vi "Station Wise Live Breakdown Status.vi"() -> ()   [LabVIEW 2017]
uses:
  Controls/Station_wise_live_breakdown_loop.ctl
  Controls/station_wise_loop_data.ctl
  <vilib>/addons/database/Connection.llb/Conn ObjectReference.ctl
  <vilib>/addons/database/Connection.llb/DB Tools Open Connec (Path).vi
  <vilib>/addons/database/Connection.llb/Conn Execute.vi
  <vilib>/addons/database/Recordset.llb/Rec Fetch Recordset Data (R).vi
  <vilib>/addons/database/Recordset.llb/Rec Destroy - Connection.vi
  Globle/Global 1.vi
  <vilib>/addons/database/NI_Database_API.lvlib
panel:
  out "ACTUAL  PLC COUNT":i32
  out "MACHINE 13":string
  out "Recipe Number":i32
  out "Product Code/":cluster{string, "ACTUAL  PLC COUNT":i32}[](array[cluster])
  out "Station Name":string[](array[string])
  out "Station Number":string[](array[string])
  out "Product List 2":string[][](array[string])
  out "appended path 2":path
  out "Product List":string[][](array[string])
  in  "Close":bool
  out "?":T1[](array[typedef])
  out "appended array":u32[](array[numeric])
  out "Table 2":string[][](array[string])
  out "String 2":string
  out "ACTUAL  PLC COUNT 2":i32
  out "ACTUAL  PLC PRODUCT CODE 2":i32
  out "Date / Time : 4":string
  out "String":string
  out "Table":string[][](array[string])
  out "Date / Time : 3":string
  out "ALARM ARRAY":string[](array[string])
  out "ALARAM CLST REF":bool
  out "String Indicator 8":bool
  out "Shift Time stamp":timestamp[](array[timestamp]) format="%<%X>T"
  in  "error in":errorcluster
  in  "Product code":string
  out "Production Count 7":i32
  in  "Rejection count 7":i32
  in  "Tab Control":T2(tab)
  out "Display 3":T3
  out "Display 1":T4
  out "Display 2":T3
  out "Display 4":T3
  out "Display 5":T3
  out "Display 6":T3
  out "Display 7":T3
  out "Display 8":T3
  out "Display 9":T3
  out "Display 10":T5
  out "MACHINE 12":cluster{"M1.1 8":bool, "M1.1 9":bool}
  out "MACHINE 11":string
  out "MACHINE 10":string
  out "MACHINE 8":string
  out "MACHINE 7":string
  out "MACHINE 6":string
  out "MACHINE 5":string
  out "MACHINE 4":string
  out "MACHINE 3":string
  out "MACHINE 2":string
  out "MACHINE 1":string
  out "MACHINE 8":T6
  out "MACHINE 7":T6
  out "MACHINE 6":T6
  out "MACHINE 5":T6
  out "MACHINE 4":T6
  out "MACHINE 3":T6
  out "MACHINE 2":T6
  out "Autonomous Check Points Press":T7
  out "MACHINE 1":T6
  out "MACHINE 9":T6
  out "MACHINE 10":T6
  out "Autonomous Check Points Oven":cluster{"ALARAM 1":bool}
  out "OVEN STATUS AUTONOMOUS":T8
  out "10":T9 caption="500T-1345678998uiyfghbu" {"PRESSURE_2nd" format="%#_g bar"; "PRESSURE_1st" format="%#_g bar"; "HOLDING_TIME" format="%#_g Sec"; "MR_RETURN_TIME" format="%#_g Sec"}
  out "9":T9 caption="500T-1" {"PRESSURE_2nd" format="%#_g bar"; "PRESSURE_1st" format="%#_g bar"; "HOLDING_TIME" format="%#_g Sec"; "MR_RETURN_TIME" format="%#_g Sec"}
  out "8":T9 caption="400T-4" {"PRESSURE_2nd" format="%#_g bar"; "PRESSURE_1st" format="%#_g bar"; "HOLDING_TIME" format="%#_g Sec"; "MR_RETURN_TIME" format="%#_g Sec"}
  out "6":T9 caption="250T-3" {"PRESSURE_2nd" format="%#_g bar"; "PRESSURE_1st" format="%#_g bar"; "HOLDING_TIME" format="%#_g Sec"; "MR_RETURN_TIME" format="%#_g Sec"}
  out "5":T9 caption="400T-1" {"PRESSURE_2nd" format="%#_g bar"; "PRESSURE_1st" format="%#_g bar"; "HOLDING_TIME" format="%#_g Sec"; "MR_RETURN_TIME" format="%#_g Sec"}
  out "4":T9 caption="400T-2" {"PRESSURE_2nd" format="%#_g bar"; "PRESSURE_1st" format="%#_g bar"; "HOLDING_TIME" format="%#_g Sec"; "MR_RETURN_TIME" format="%#_g Sec"}
  out "1":T9 caption="150T-1" {"PRESSURE_2nd" format="%#_g bar"; "PRESSURE_1st" format="%#_g bar"; "HOLDING_TIME" format="%#_g Sec"; "MR_RETURN_TIME" format="%#_g Sec"}
  out "2":T9 caption="250T-2" {"PRESSURE_2nd" format="%#_g bar"; "PRESSURE_1st" format="%#_g bar"; "HOLDING_TIME" format="%#_g Sec"; "MR_RETURN_TIME" format="%#_g Sec"}
  out "3":T9 caption="400T-3" {"PRESSURE_2nd" format="%#_g bar"; "PRESSURE_1st" format="%#_g bar"; "HOLDING_TIME" format="%#_g Sec"; "MR_RETURN_TIME" format="%#_g Sec"}
  out "7":T9 caption="250T-4" {"PRESSURE_2nd" format="%#_g bar"; "PRESSURE_1st" format="%#_g bar"; "HOLDING_TIME" format="%#_g Sec"; "MR_RETURN_TIME" format="%#_g Sec"}
  out "1 5":T10 caption="400T-4 OVEN" {"Heating_time" format="%#_g Sec"; "Bottom_zone_8" format="%#_g °C"; "Bottom_zone_7" format="%#_g °C"; "Bottom_zone_6" format="%#_g °C"; "Bottom_zone_5" format="%#_g °C"; "Bottom_zone_4" format="%#_g °C"; "Bottom_zone_3" format="%#_g °C"; "Bottom_zone_2" format="%#_g °C"; "Bottom_zone_1" format="%#_g °C"; "Top_zone_8" format="%#_g °C"; "Top_zone_7" format="%#_g °C"; "Top_zone_6" format="%#_g °C"; "Top_zone_5" format="%#_g °C"; "Top_zone_4" format="%#_g °C"; "Top_zone_3" format="%#_g °C"; "Top_zone_2" format="%#_g °C"; "Top_zone_1" format="%#_g °C"}
  out "1 4":T10 caption="400T-3 OVEN" {"Heating_time" format="%#_g Sec"; "Bottom_zone_8" format="%#_g °C"; "Bottom_zone_7" format="%#_g °C"; "Bottom_zone_6" format="%#_g °C"; "Bottom_zone_5" format="%#_g °C"; "Bottom_zone_4" format="%#_g °C"; "Bottom_zone_3" format="%#_g °C"; "Bottom_zone_2" format="%#_g °C"; "Bottom_zone_1" format="%#_g °C"; "Top_zone_8" format="%#_g °C"; "Top_zone_7" format="%#_g °C"; "Top_zone_6" format="%#_g °C"; "Top_zone_5" format="%#_g °C"; "Top_zone_4" format="%#_g °C"; "Top_zone_3" format="%#_g °C"; "Top_zone_2" format="%#_g °C"; "Top_zone_1" format="%#_g °C"}
  out "1 3":T10 caption="400T-2 OVEN" {"Heating_time" format="%#_g Sec"; "Bottom_zone_8" format="%#_g °C"; "Bottom_zone_7" format="%#_g °C"; "Bottom_zone_6" format="%#_g °C"; "Bottom_zone_5" format="%#_g °C"; "Bottom_zone_4" format="%#_g °C"; "Bottom_zone_3" format="%#_g °C"; "Bottom_zone_2" format="%#_g °C"; "Bottom_zone_1" format="%#_g °C"; "Top_zone_8" format="%#_g °C"; "Top_zone_7" format="%#_g °C"; "Top_zone_6" format="%#_g °C"; "Top_zone_5" format="%#_g °C"; "Top_zone_4" format="%#_g °C"; "Top_zone_3" format="%#_g °C"; "Top_zone_2" format="%#_g °C"; "Top_zone_1" format="%#_g °C"}
  out "1 2":T10 caption="400T-1 OVEN" {"Heating_time" format="%#_g Sec"; "Bottom_zone_8" format="%#_g °C"; "Bottom_zone_7" format="%#_g °C"; "Bottom_zone_6" format="%#_g °C"; "Bottom_zone_5" format="%#_g °C"; "Bottom_zone_4" format="%#_g °C"; "Bottom_zone_3" format="%#_g °C"; "Bottom_zone_2" format="%#_g °C"; "Bottom_zone_1" format="%#_g °C"; "Top_zone_8" format="%#_g °C"; "Top_zone_7" format="%#_g °C"; "Top_zone_6" format="%#_g °C"; "Top_zone_5" format="%#_g °C"; "Top_zone_4" format="%#_g °C"; "Top_zone_3" format="%#_g °C"; "Top_zone_2" format="%#_g °C"; "Top_zone_1" format="%#_g °C"}
  out "1 8":T11 caption="500T-1 OVEN" {"Bottom Zone\ntemperature" format="%#_g °C"; "Heating_time" format="%#_g Sec"; "Top Zone\ntemperature" format="%#_g °C"}
  out "1 7":T12 caption="250T-1 OVEN" {"Heating_time" format="%#_g Sec"; "Bottom_zone_3" format="%#_g °C"; "Bottom_zone_2" format="%#_g °C"; "Bottom_zone_1" format="%#_g °C"; "Top_zone_3" format="%#_g °C"; "Top_zone_2" format="%#_g °C"; "Top_zone_1" format="%#_g °C"}
  out "1 6":T10 caption="400T-5 OVEN" {"Heating_time" format="%#_g Sec"; "Bottom_zone_8" format="%#_g °C"; "Bottom_zone_7" format="%#_g °C"; "Bottom_zone_6" format="%#_g °C"; "Bottom_zone_5" format="%#_g °C"; "Bottom_zone_4" format="%#_g °C"; "Bottom_zone_3" format="%#_g °C"; "Bottom_zone_2" format="%#_g °C"; "Bottom_zone_1" format="%#_g °C"; "Top_zone_8" format="%#_g °C"; "Top_zone_7" format="%#_g °C"; "Top_zone_6" format="%#_g °C"; "Top_zone_5" format="%#_g °C"; "Top_zone_4" format="%#_g °C"; "Top_zone_3" format="%#_g °C"; "Top_zone_2" format="%#_g °C"; "Top_zone_1" format="%#_g °C"}
  out "error out":errorcluster
  # "CLUSTER REFRENCE"
  # "Station Wise Live Status"
  # "Communication"
  # "1st screen\n\n5 10.0.0.73\n4 10.0.0.71\n3 10.0.0.69\n7 10.0.0.61"
  # "2nd Screen\n\n8 10.0.0.63\n9 10.0.0.75\n1 10.0.0.67"
  # "Safety"
  # "Startup/Setup"
  # "1236 684"
  # "500t1 ,250-2,400-3,400-2,400-1,250-3,400-4,400-5---> PRESS\n400-1,400-2,400-3,400-4,400-5,250-1,500-1--->OVEN"
  # "1366*768"
  # "500t1 ,250-2,  400-3,400-2,400-1,250-3,400-4,400-5   ,  NA   ---> PRESS\n500-1,    NA,   400-3,400-2,400-1,   NA,    400-4,400-5, 250-1--->OVEN"
  # "Raw Material Not Available"
  # "Under Maintenance"
  # "Under Quality Review"
  # "Parameter OutOff Range"
  # "Production Recording System"
  # "Machine Under Maintanance"
  # "Product Name"
  # "Product Name"
  # "Product Name"
  # "Product Name"
  # "Product Name"
  # "Product Name"
  # "Production Recording System"
  # "Machine Under Maintanance"
  # "Product Name"
  # "Product Name"
  # "Product Name"
  # "Communication:-"
  # "Autonomous Maintanence Checksheet"
  # "T.F. Process Parameter Monitoring"
  # "Oven Process Parameter Monitoring"
  # "Machine Under Maintanance"
  # "Oven Process Parameter Monitoring"
  # "Machine Under Maintanance"
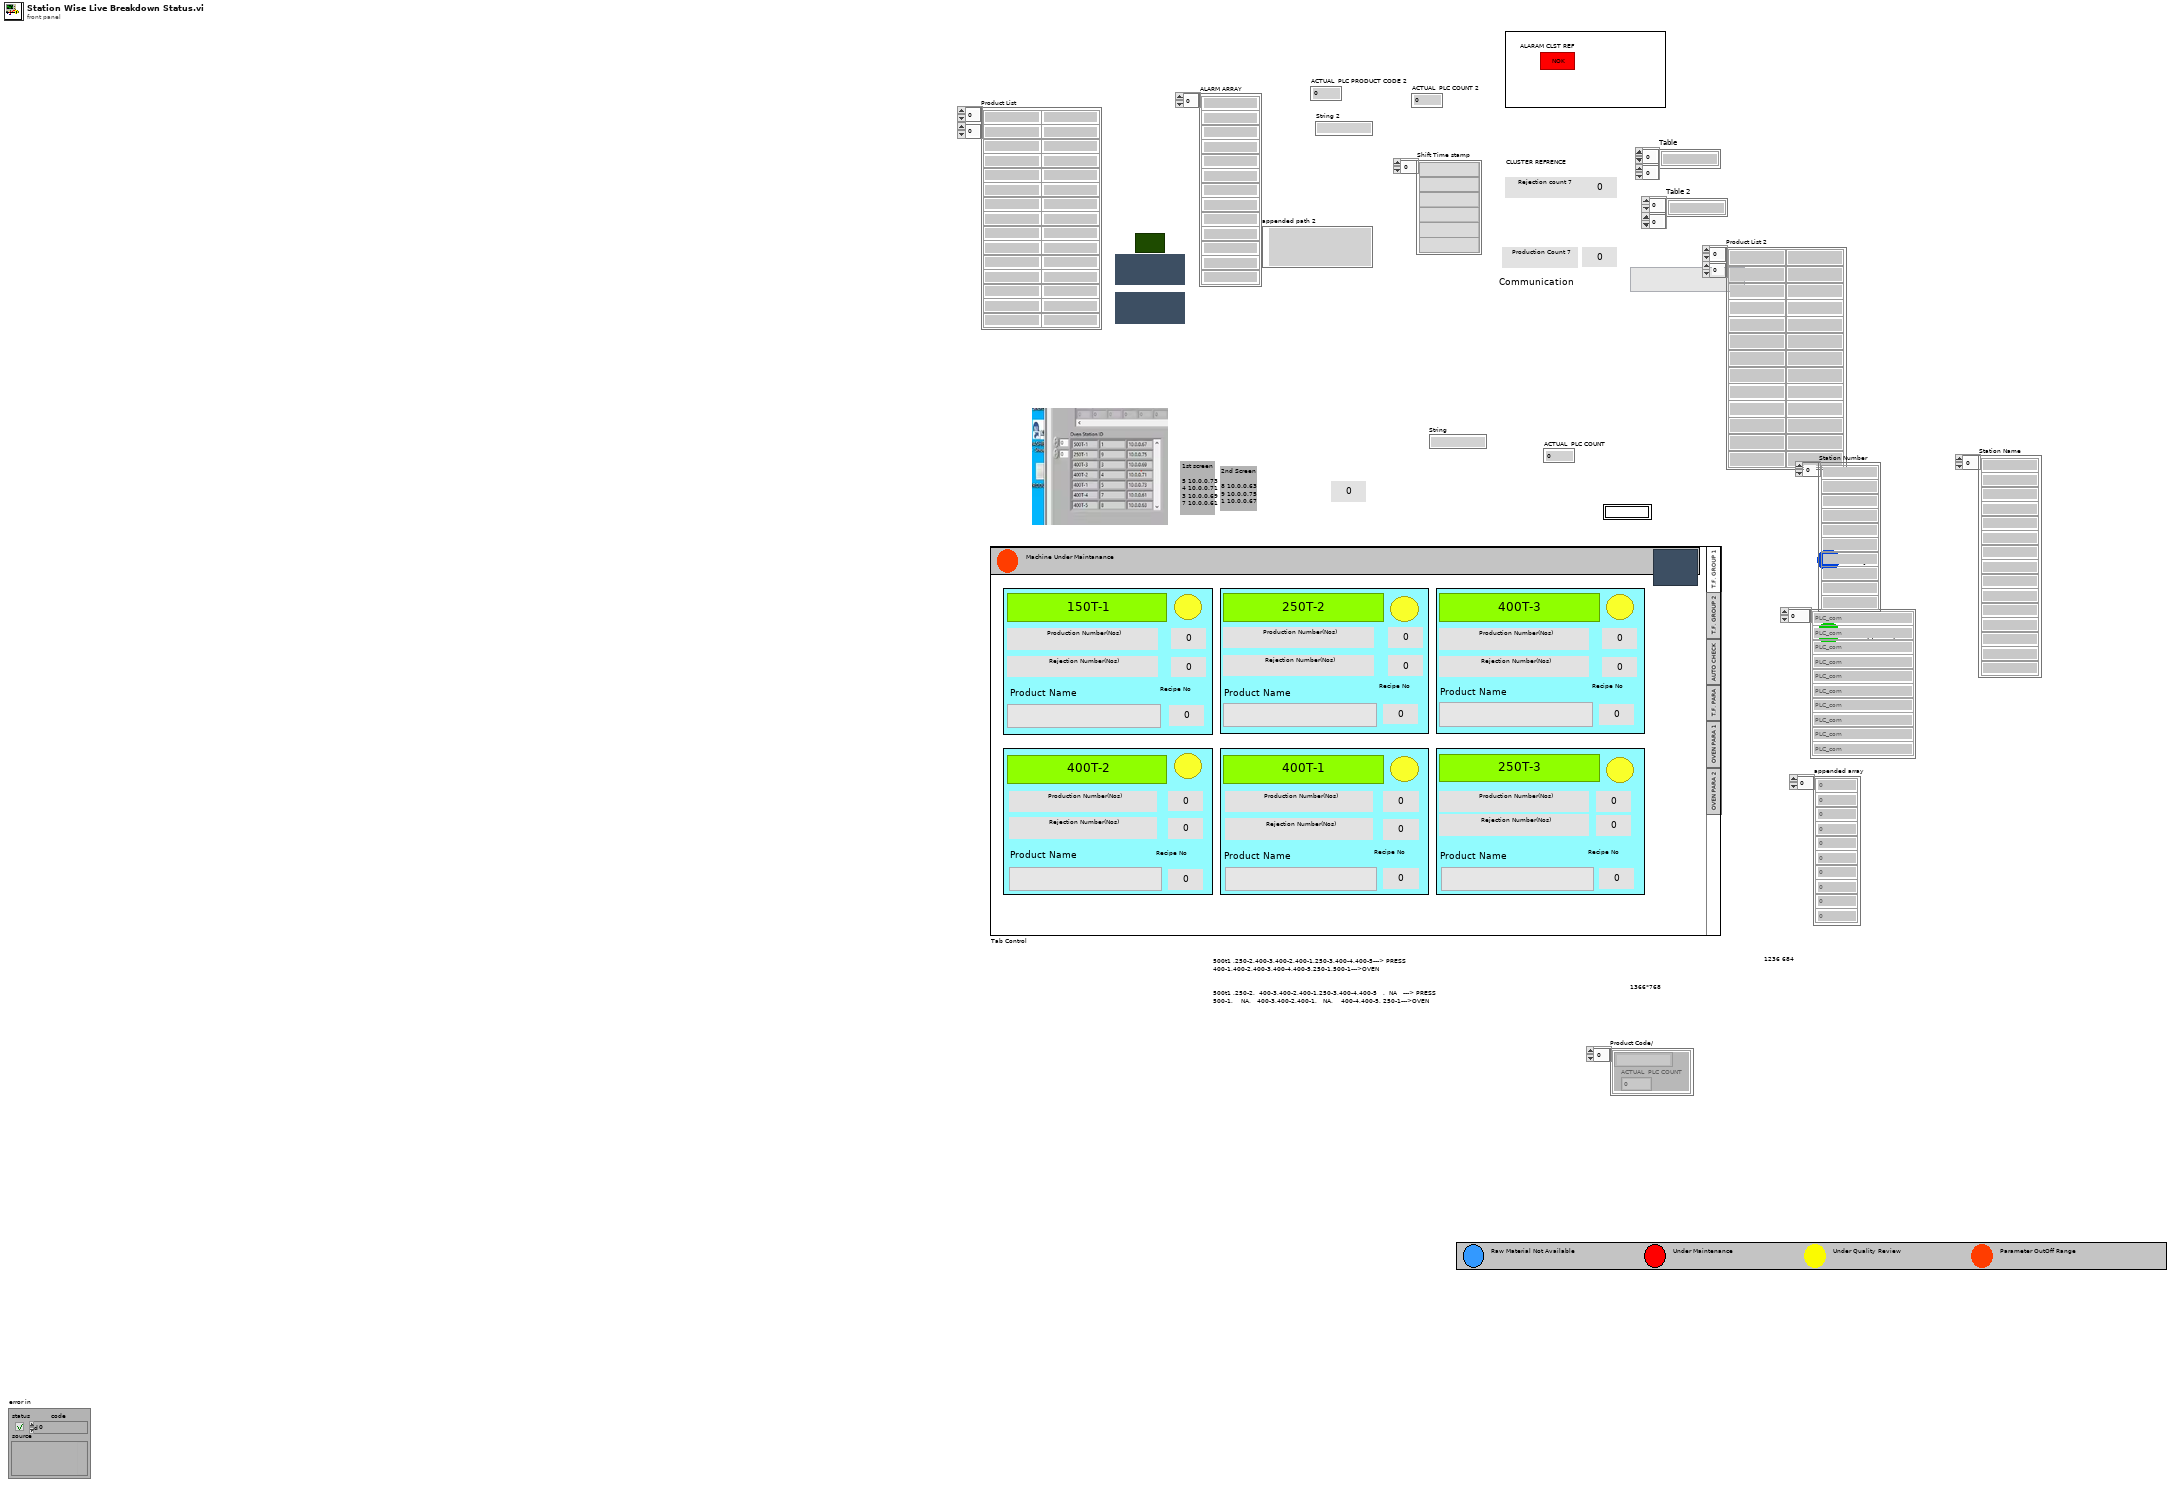
[diagram p1: front panel]
types:
  T1 = typedef "Station_wise_live_breakdown_loop.ctl" = enum16{"Int_3", "Break_down", "Rejection_count", "STOP", "BUTTON_SWITCH", "Init_2", "Alaram_stat", "Product_count", "PLC_com", "Init", "Oven_Reading"}
  T2 = enum32{"T.F. GROUP 1", "T.F. GROUP 2", "AUTO CHECK", "T.F. PARA", "OVEN PARA 1", "OVEN PARA 2"}
  T3 = cluster{"Status 10":cluster{"S":bool, "l":bool, "M":bool, "Q":bool, "P":bool}, "Station 3":bool, "Production Number(Nos)":i32, "Rejection Number(Nos)":i32, "Press COM 1":bool, "Product code 10":string, "Recipe No":i32}
  T4 = cluster{"Status 10":cluster{"S":bool, "l":bool, "M":bool, "Q":bool, "P":bool}, "Station Name":bool, "Production Number(Nos)":i32, "Rejection Number(Nos)":i32, "Press COM 1":bool, "Product code 10":string, "Recipe No":i32}
  T5 = cluster{"Status 10":cluster{"S":bool, "l":bool, "M":bool, "Q":bool, "P":bool}, "Station 3":bool, "Production\nCount 3":i32, "Rejection count 3":i32, "String Indicator 3":bool, "Product code 10":string}
  T6 = cluster{"M1.1":bool, "M1.1 2":bool, "M1.1 3":bool, "M1.1 4":bool, "M1.1 5":bool, "M1.1 6":bool, "M1.1 7":bool, "M1.1 8":bool, "M1.1 9":bool}
  T7 = cluster{"ALARAM 1":bool, "ALARAM 2":bool, "ALARAM 3":bool, "ALARAM 4":bool, "ALARAM 5":bool, "ALARAM 6":bool, "ALARAM 7":bool}
  T8 = cluster{"500T-1":bool, "M1.1 7":bool, "400T-3":bool, "400T-2":bool, "400T-1":bool, "M1.1 7":bool, "M1.1 6":bool, "M1.1 10":bool, "M1.1 11":bool}
  T9 = cluster{"MR_RETURN_TIME":dbl, "HOLDING_TIME":dbl, "PRESSURE_1st":dbl, "PRESSURE_2nd":dbl}
  T10 = cluster{"400T-2 OVEN COM":bool, "Station Name 2":bool, "Top_zone_1":dbl, "Top_zone_2":dbl, "Top_zone_3":dbl, "Top_zone_4":dbl, "Top_zone_5":dbl, "Top_zone_6":dbl, "Top_zone_7":dbl, "Top_zone_8":dbl, "Bottom_zone_1":dbl, "Bottom_zone_2":dbl, "Bottom_zone_3":dbl, "Bottom_zone_4":dbl, "Bottom_zone_5":dbl, "Bottom_zone_6":dbl, "Bottom_zone_7":dbl, "Bottom_zone_8":dbl, "Heating_time":dbl}
  T11 = cluster{"400T-2 OVEN COM":bool, "Station Name 2":bool, "Top Zone\ntemperature":dbl, "Bottom Zone\ntemperature":dbl, "Heating_time":dbl}
  T12 = cluster{"400T-2 OVEN COM":bool, "Station Name 2":bool, "Top_zone_1":dbl, "Top_zone_2":dbl, "Top_zone_3":dbl, "Bottom_zone_1":dbl, "Bottom_zone_2":dbl, "Bottom_zone_3":dbl, "Heating_time":dbl}
  T13 = typedef "station_wise_loop_data.ctl" = cluster{"Product List":string[][], "SQL reference":T14, "Indicator refrence":refnum<vi>[], "Station Number":string[], "Shift Time stamp":timestamp[], "Com Status Station":string[], "ALARAM INDICATOR REF":refnum<vi>[], "Reading":refnum<vi>[], "Read Parameteres":string[][], "Station Name":string[], "Oven Read Parameteres":string[][]}
  T14 = typedef "NI_Database_API.lvlib/Conn ObjectReference.ctl" = refnum<k1>
  T15 = enum32{"invalid app kind", "Development System", "Run Time System", "Student Edition", "Embedded LabVIEW", "Evaluation", "Custom"}
  T16 = typedef "NI_Database_API.lvlib/Rec ObjectReference.ctl" = refnum<k1>
  T17 = enum32{"T.F. GROUP 1", "T.F. GROUP 2", "AUTO CHECK", "T.F. PARA", "OVEN PARA 1", "OVEN PARA 2"}[]
  T18 = cluster{"[0]":dbl, "[1]":dbl, "[2]":dbl, "[3]":dbl}
  T19 = cluster{"[0]":bool, "[1]":bool, "[2]":bool, "[3]":bool, "[4]":bool}
  T20 = cluster{"array[0]":bool, "array[1]":bool, "array[2]":bool, "array[3]":bool, "array[4]":bool}
  T21 = cluster{"[0]":bool, "[1]":bool, "[2]":bool, "[3]":bool, "[4]":bool, "[5]":bool, "[6]":bool, "[7]":bool, "[8]":bool}
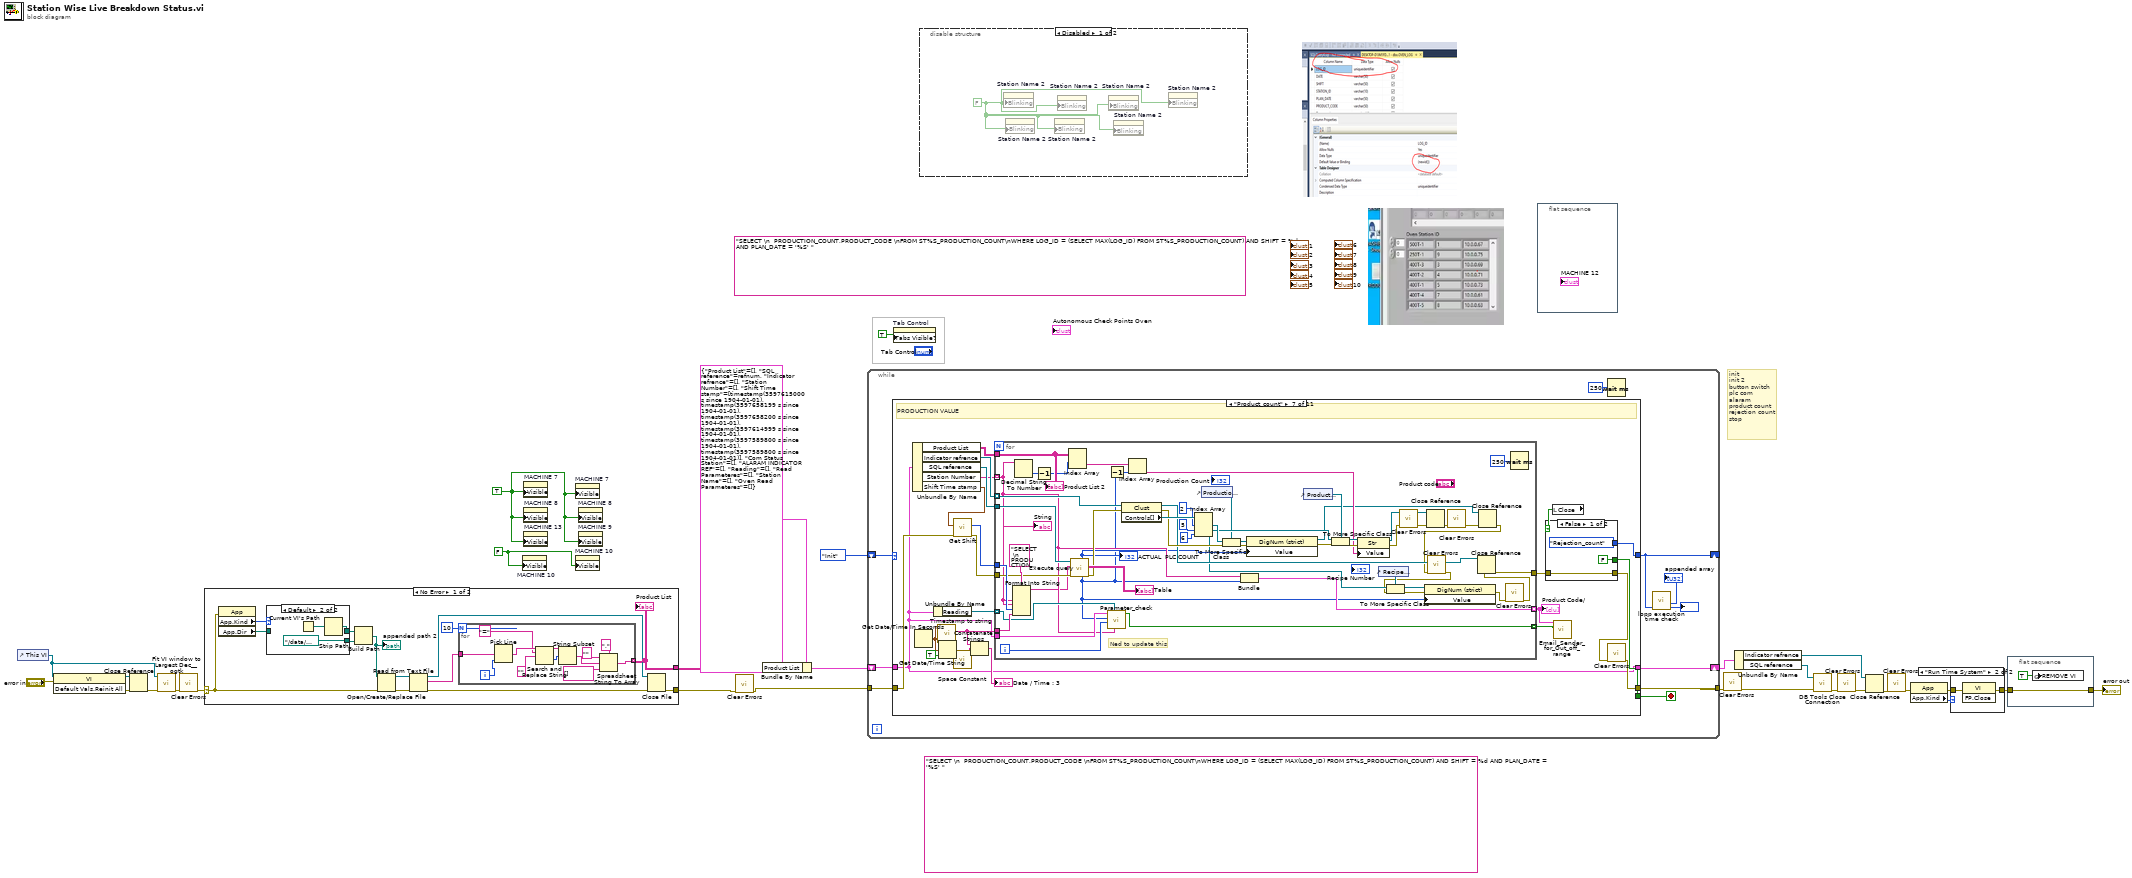
[diagram p0: block diagram]
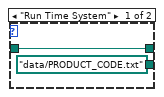
[diagram p4: hidden frame]
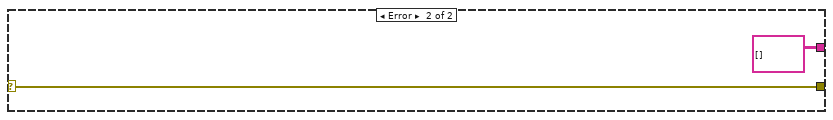
[diagram p5: hidden frame]
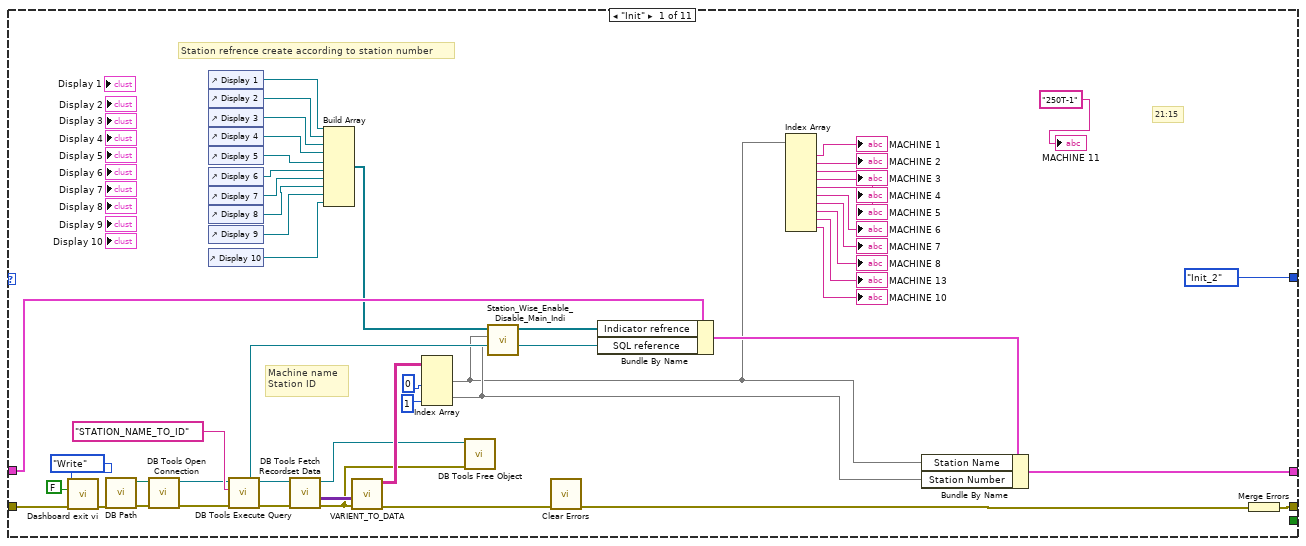
[diagram p6: hidden frame]
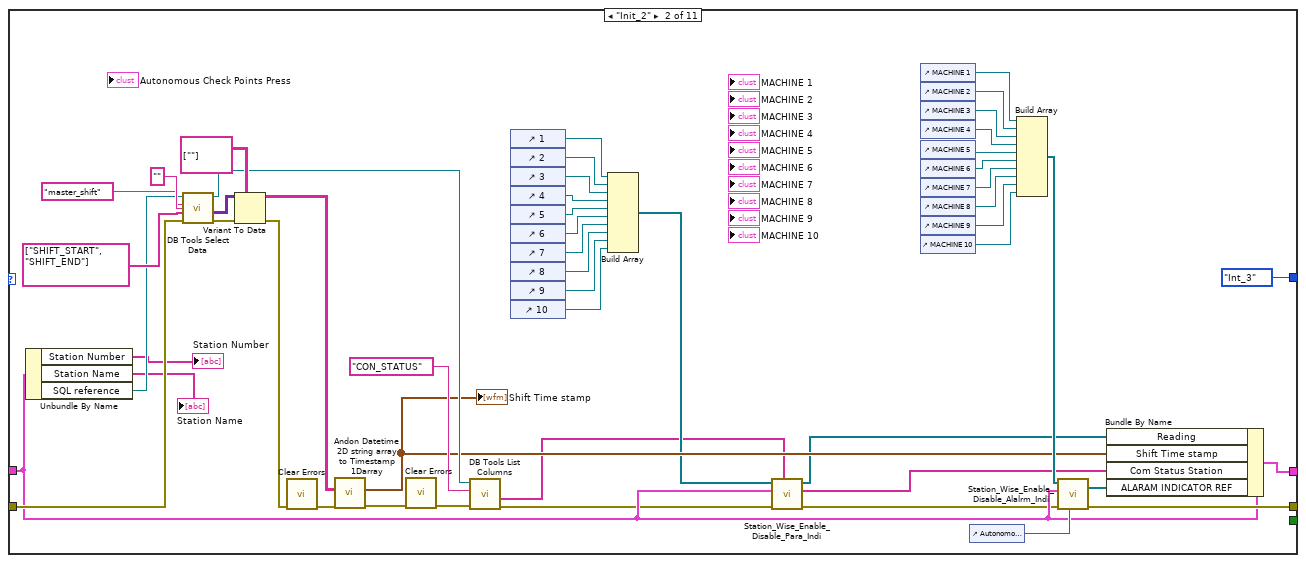
[diagram p7: hidden frame]
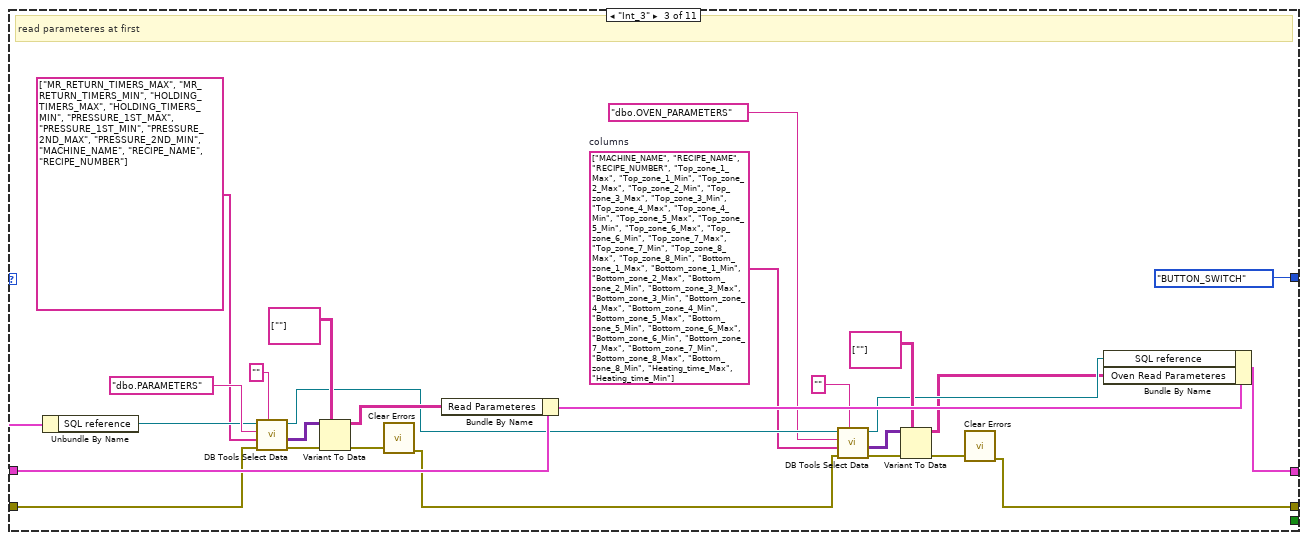
[diagram p8: hidden frame]
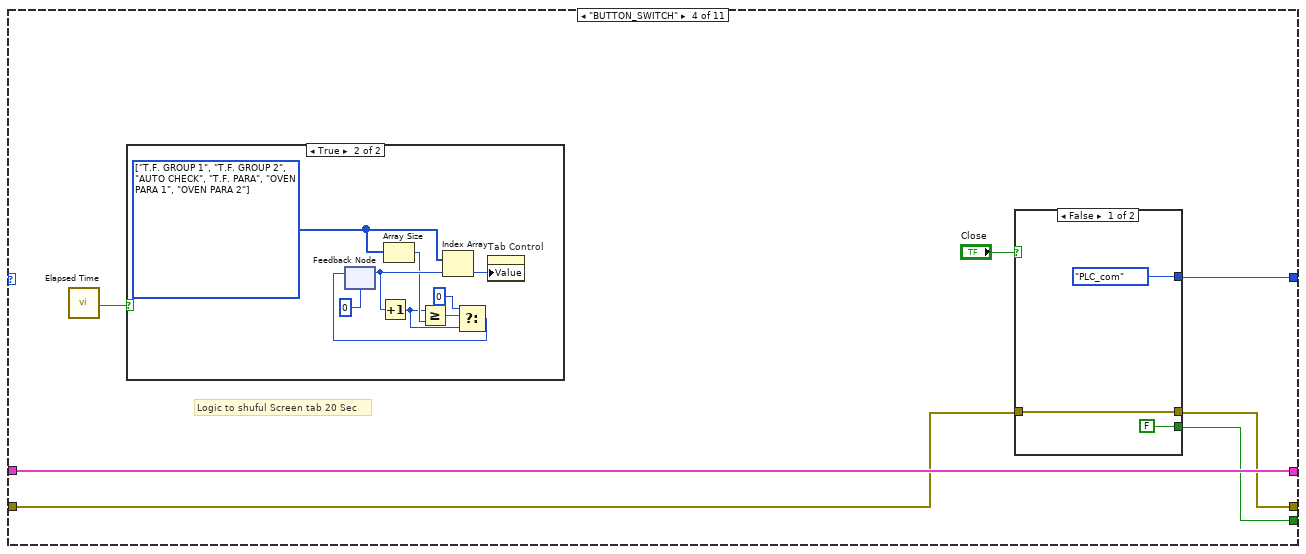
[diagram p9: hidden frame]
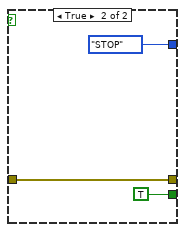
[diagram p11: hidden frame]
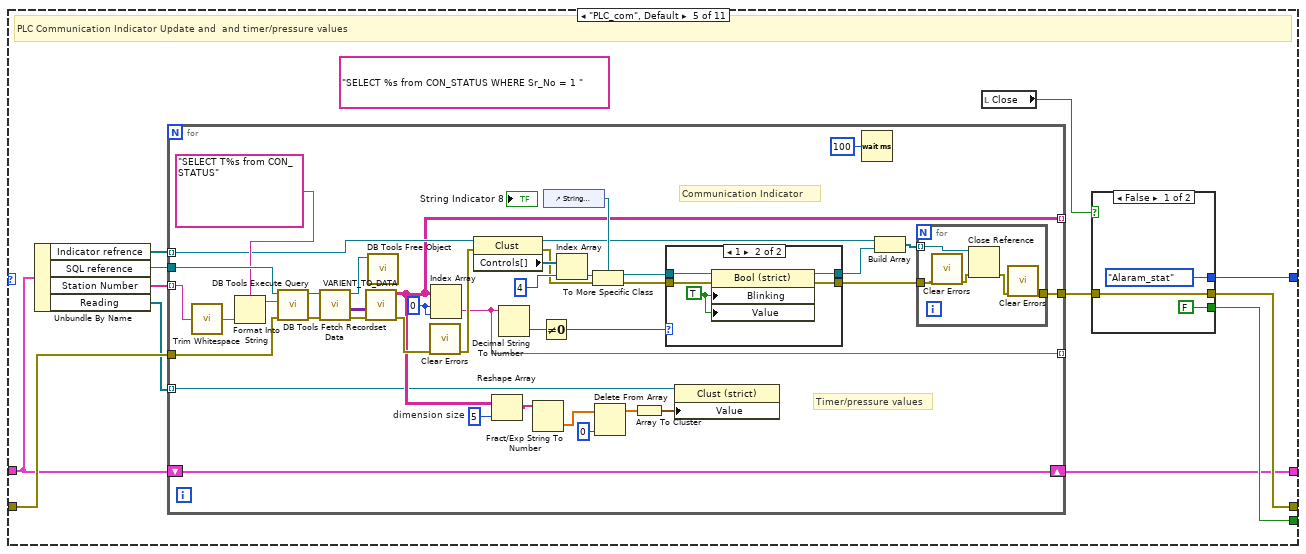
[diagram p12: hidden frame]
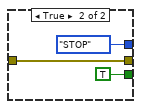
[diagram p13: hidden frame]
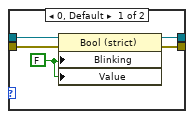
[diagram p14: hidden frame]
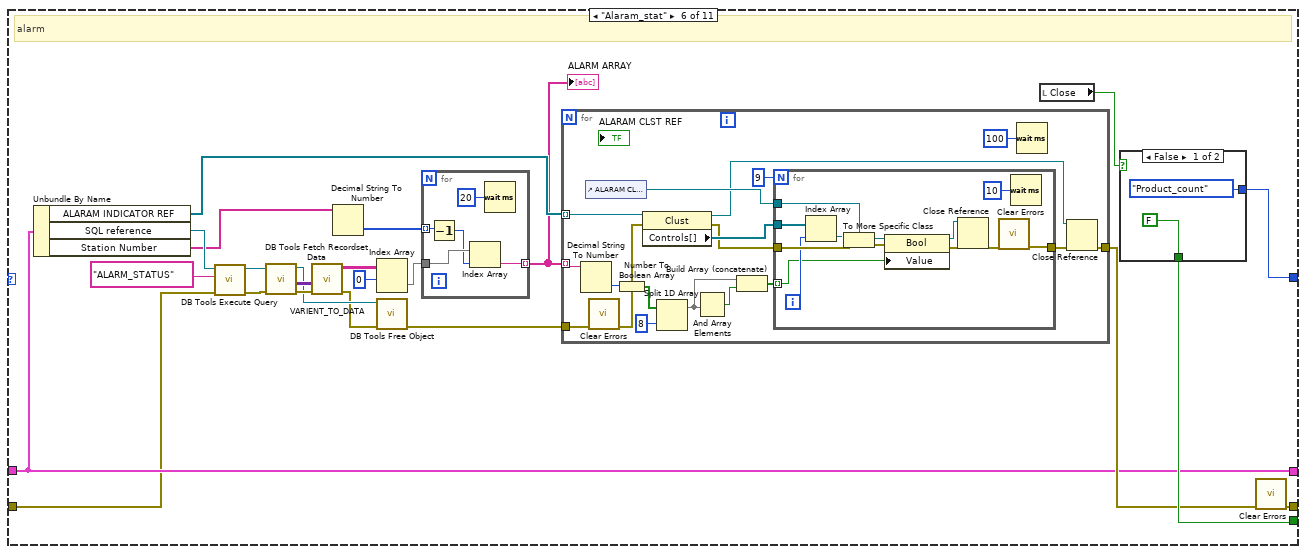
[diagram p15: hidden frame]
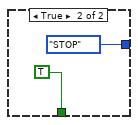
[diagram p16: hidden frame]
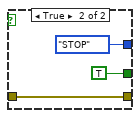
[diagram p17: hidden frame]
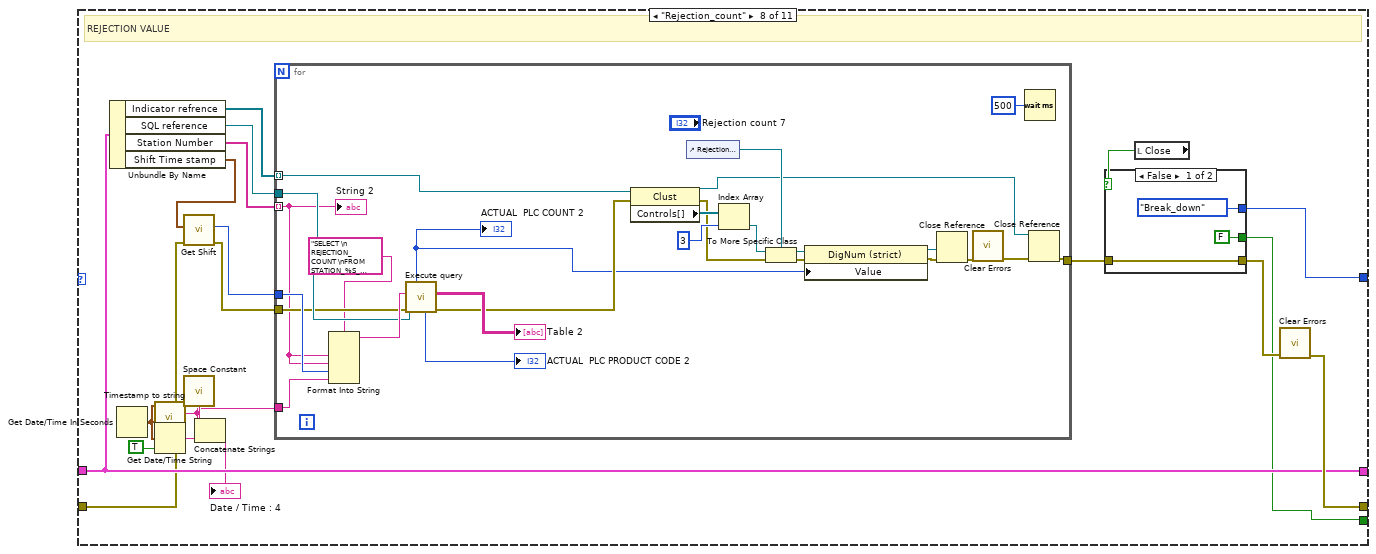
[diagram p18: hidden frame]
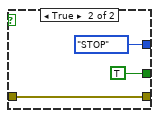
[diagram p19: hidden frame]
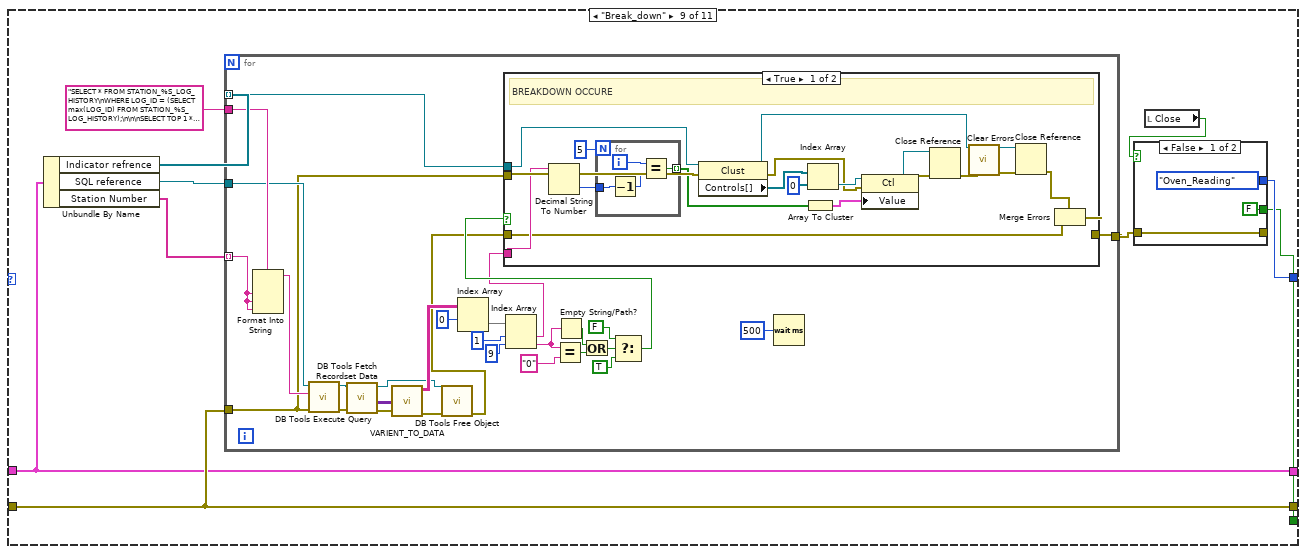
[diagram p20: hidden frame]
diagram:
  (unwired) "SELECT \n  PRODUCTION_COUNT,PRODUCT_CODE \nFROM ST%S_PRODUCTION_COUNT\nWHERE LOG_ID = (SELECT MAX(LOG_ID) FROM ST%S_PRODUCTION_COUNT) AND SHIFT = %d AND PLAN_DATE = '%S' " ("SQL query")
  (unwired) "SELECT \n  PRODUCTION_COUNT,PRODUCT_CODE \nFROM ST%S_PRODUCTION_COUNT\nWHERE LOG_ID = (SELECT MAX(LOG_ID) FROM ST%S_PRODUCTION_COUNT) AND SHIFT = %d AND PLAN_DATE = '%S' " ("SQL query")
  w5 = FALSE
  w19 = TRUE
  # "init\ninit 2\nbutton switch\nplc com\nalaram\nproduct count\nrejection count\nstop"
  n1 = control-ref of="This VI"() -> (w2:refnum<vi>)
  n2 = invoke class="VI" method="Default Vals.Reinit All"(reference=w2, error in="error in") -> (reference out=w8:refnum<vi>, error out=w7:errorcluster)  [unwired: 1 in, 1 out]
  n3 = Close Reference(reference=w8, error in (no error)=w7) -> (error out=w4:errorcluster)
  n4 = call <userlib>:"Fit VI window to Largest Dec__ogtk.vi"("error in (no error)"=w4, "VI Ref (calling VI)"=w2) -> ("error out"=w3:errorcluster)  [unwired: 4 in, 1 out]
  n5 = call <vilib>:"Clear Errors.vi"("error in (no error)"=w3) -> ("error out"=w1:errorcluster)  [unwired: 5 in, 1 out]
  n6 = case shown="No Error" w1 {
    selector: w1 -> [w30 w62]
    tunnel: [w34 w62] -> w10
    tunnel: [w31 string[][] [] ("delimiter (Tab)")] -> w28
    frame No Error {
      n7 = property class="App"(error in=w30) -> ("App.Kind"=w43:T15, "App.Dir"=w42:path)  [unwired: 1 in, 2 out]
      n8 = case shown="Default" w43 {
        tunnel: w42 -> [w57 _]
        tunnel: [path "data/PRODUCT_CODE.txt" ("path") path "../data/PRODUCT_CODE.txt" ("path")] -> w40
        tunnel: [w57 w58] -> w39
        frame "Run Time System" {
        }
        frame Default {
          n9 = Current VI's Path() -> (path=w59:path)
          n10 = Strip Path(path=w59) -> (stripped path=w58:path)  [unwired: 1 out]
        }
      }
      n11 = Build Path(base path=w39, name or relative path=w40) -> (appended path=w41:path)
      "appended path 2" <- w41
      n12 = Open/Create/Replace File(file path (use dialog)=w41, error in=w30) -> (refnum out=w38:refnum<file>, error out=w37:errorcluster)  [unwired: 4 in, 1 out]
      n13 = Read from Text File(file (use dialog)=w38, error in=w37) -> (refnum out=w35:refnum<file>, text=w33:string, error out=w36:errorcluster)  [unwired: 2 in, 1 out]
      n14 = for {
        N: 10 -> [_]
        tunnel: w33 -> [w46]
        tunnel: [w44] -> w31 mode=indexing
        i -> [w47]
        n15 = Pick Line(multi-line string=w46, line index=w47) -> (output string=w48:string)  [unwired: 1 in]
        n16 = Search and Replace String(input string=w48, search string="=" ("format string"), replace string="" ("search string")) -> (result string=w50:string, offset past replacement=w51:i32)  [unwired: 5 in, 2 out]
        n17 = String Subset(string=w50, offset (0)=w51) -> (substring=w49:string)  [unwired: 1 in]
        n18 = Spreadsheet String To Array(delimiter (Tab)=",", format string="", spreadsheet string=w49, array type (2D Dbl)=string[] [] ("delimiter (Tab)")) -> (array=w44:string[])
      }
      "Product List" <- w31
      n19 = Close File(refnum=w35, error in=w36) -> (error out=w34:errorcluster)  [unwired: 1 out]
    }
    frame Error {
    }
  }
  n20 = property on="MACHINE 10" class="Str"("Visible"=w5) -> ()  [unwired: 2 in, 2 out]
  n21 = property on="MACHINE 7" class="Str"("Visible"=w19) -> ()  [unwired: 2 in, 2 out]
  n22 = property on="MACHINE 8" class="Str"("Visible"=w19) -> ()  [unwired: 2 in, 2 out]
  n23 = property on="MACHINE 13" class="Str"("Visible"=w19) -> ()  [unwired: 2 in, 2 out]
  n24 = property on="MACHINE 7" class="Clust"("Visible"=w19) -> ()  [unwired: 2 in, 2 out]
  n25 = property on="MACHINE 10" class="Clust"("Visible"=w5) -> ()  [unwired: 2 in, 2 out]
  n26 = property on="MACHINE 8" class="Clust"("Visible"=w19) -> ()  [unwired: 2 in, 2 out]
  n27 = property on="MACHINE 9" class="Clust"("Visible"=w19) -> ()  [unwired: 2 in, 2 out]
  n28 = call <vilib>:"Clear Errors.vi"("error in (no error)"=w10) -> ("error out"=w9:errorcluster)  [unwired: 5 in, 1 out]
  n29 = Bundle By Name(cluster=T13 {"Product List"=[], "SQL reference"=refnum, "Indicator refrence"=[], "Station Number"=[], "Shift Time stamp"=[timestamp(3597615000 s since 1904-01-01), timestamp(3597658199 s since 1904-01-01), timestamp(3597658200 s since 1904-01-01), timestamp(3597614999 s since 1904-01-01), timestamp(3597589800 s since 1904-01-01), timestamp(3597589800 s since 1904-01-01)], "Com Status Station"=[], "ALARAM INDICATOR REF"=[], "Reading"=[], "Read Parameteres"=[], "Station Name"=[], "Oven Read Parameteres"=[]}, "Product List"=w28) -> (w27:T13)
  n30 = while {
    tunnel: w9 -> [w71]
    tunnel: [w70] -> w11
    shift-right: [w69] -> w23
    shift-left: w27 -> [w68]
    shift-right: [w65] -> _
    shift-left: Station_wise_live_breakdown_loop."Init" -> [w72]
    stop <- w67 stop-if-true
    n31 = case shown="\"Product_count\"" w72 {
      tunnel: w71 -> [w109 w163 w187 w201 w229 w294 w374 w453 w501 w642 w649]
      tunnel: w68 -> [w115 w128 w189 w205 w222 w295 w358 w455 w500 w589 w655]
      tunnel: [w95 w143 w178 w200 w226 w314 w376 w456 w501 w641 w650] -> w70
      tunnel: [w93 w151 w185 w205 w221 w295 w358 w455 w500 w589 w655] -> w69
      tunnel: [Station_wise_live_breakdown_loop."Init_2" Station_wise_live_breakdown_loop."Int_3" Station_wise_live_breakdown_loop."BUTTON_SWITCH" w204 w225 w298 w361 w441 w493 Station_wise_live_breakdown_loop."BUTTON_SWITCH" Station_wise_live_breakdown_loop."STOP"] -> w65
      tunnel: [_ _ _ w202 w224 w297 w360 w440 w492 _ TRUE] -> w67
      frame "Init" {
        # "21:15"
        # "Machine name\nStation ID"
        # "Station refrence create according to station number"
        n32 = call "Dashboard exit vi.vi"("error in (no error)"=w109, "Exit in"=FALSE, "Enum"=enum16{"Write", "Read"}."Write") -> ("error out"=w113:errorcluster)  [unwired: 7 in, 1 out]
        n33 = call "DB Path.vi"("error in"=w113) -> ("error out"=w112:errorcluster, "DB Path"=w114:path)  [unwired: 9 in]
        n34 = call-poly <vilib>:"DB Tools Open Connection.vi"("error in (no error)"=w112, "connection information"=w114) -> ("error out"=w105:errorcluster, "connection reference"=w104:T14)  [unwired: 6 in]
        n35 = control-ref of="Display 1"() -> (w116:refnum<vi>)
        n36 = control-ref of="Display 2"() -> (w117:refnum<vi>)
        n37 = control-ref of="Display 3"() -> (w118:refnum<vi>)
        n38 = control-ref of="Display 4"() -> (w119:refnum<vi>)
        n39 = control-ref of="Display 5"() -> (w120:refnum<vi>)
        n40 = control-ref of="Display 6"() -> (w121:refnum<vi>)
        n41 = control-ref of="Display 7"() -> (w81:refnum<vi>)
        n42 = control-ref of="Display 8"() -> (w80:refnum<vi>)
        n43 = control-ref of="Display 9"() -> (w79:refnum<vi>)
        n44 = control-ref of="Display 10"() -> (w78:refnum<vi>)
        n45 = call-poly <vilib>:"DB Tools Execute Query.vi"("error in (no error)"=w105, "SQL query"="STATION_NAME_TO_ID", "connection reference"=w104) -> ("error out"=w107:errorcluster, "recordset reference"=w108:T16)  [unwired: 5 in]
        n46 = call-poly <vilib>:"DB Tools Fetch Recordset Data.vi"("error in (no error)"=w107, "recordset reference"=w108) -> ("error out"=w98:errorcluster, "recordset data"=w103:variant[][], "recordset reference out"=w99:T16)  [unwired: 3 in]
        n47 = Build Array(w116, w117, w118, w119, w120, w121, w81, w80, w79, w78) -> (w75:refnum<vi>[])
        n48 = call "VARIENT_TO_DATA.vi"("data"=w103, "error in (no error)"=w98) -> ("Table"=w100:string[][], "error out"=w97:errorcluster)  [unwired: 7 in]
        n49 = Index Array(array=w100, index (col) #1=0 ("index (row)"), index (col) #2=1 ("index (col)")) -> (element #1=w76:string[], element #2=w77:string[])  [unwired: 2 in]
        n50 = call-poly <vilib>:"DB Tools Free Object.vi"("error in (no error)"=w98, "recordset reference"=w99) -> ()  [unwired: 8 in, 2 out]
        n51 = call "Station_Wise_Enable_Disable_Main_Indi.vi"("Station number"=w77, "Station name"=w76, "appended array"=w75) -> ("Valid Indicators"=w74:refnum<vi>[])  [unwired: 7 in, 1 out]
        n52 = call <vilib>:"Clear Errors.vi"("error in (no error)"=w97) -> ("error out"=w96:errorcluster)  [unwired: 5 in, 1 out]
        n53 = Bundle By Name(cluster=w115, "Indicator refrence"=w74, "SQL reference"=w104) -> (w94:T13)
        n54 = Index Array(array=w76) -> (element #1=→"MACHINE 1":string, element #2=→"MACHINE 2":string, element #3=→"MACHINE 3":string, element #4=→"MACHINE 4":string, element #5=→"MACHINE 5":string, element #6=→"MACHINE 6":string, element #7=→"MACHINE 7":string, element #8=→"MACHINE 8":string, element #9=→"MACHINE 13":string, element #10=→"MACHINE 10":string)  [unwired: 10 in]
        n55 = Bundle By Name(cluster=w94, "Station Name"=w76, "Station Number"=w77) -> (w93:T13)
        n56 = Merge Errors(w96) -> (w95:errorcluster)
        "MACHINE 11" <- "250T-1"
      }
      frame "Init_2" {
        n57 = Unbundle By Name(w128) -> ("Station Number"=→"Station Number":string[], "Station Name"=→"Station Name":string[], "SQL reference"=w162:T14)
        n58 = call <vilib>:"DB Tools Select Data.vi"("condition"="", "error in (no error)"=w163, "columns"=string[] ["SHIFT_START", "SHIFT_END"], "table"="master_shift", "connection reference"=w162) -> ("error out"=w170:errorcluster, "data"=w168:variant[][], "connection reference out"=w159:T14)  [unwired: 1 in]
        n59 = Variant To Data(error in=w170, type=string[][] [[""]], Variant=w168) -> (data=w169:string[][], error out=w171:errorcluster)
        n60 = call <vilib>:"Clear Errors.vi"("error in (no error)"=w171) -> ("error out"=w172:errorcluster)  [unwired: 5 in, 1 out]
        n61 = call "Andon Datetime 2D string array to Timestamp 1Darray.vi"("error in (no error)"=w172, "String Array In"=w169) -> ("error out"=w161:errorcluster, "Time Stamp Out"=w141:timestamp[])  [unwired: 8 in]
        "Shift Time stamp" <- w141
        n62 = call <vilib>:"Clear Errors.vi"("error in (no error)"=w161) -> ("error out"=w158:errorcluster)  [unwired: 5 in, 1 out]
        n63 = call <vilib>:"DB Tools List Columns.vi"("error in (no error)"=w158, "table"="CON_STATUS", "connection reference"=w159) -> ("error out"=w127:errorcluster, "columns"=w123:string[])  [unwired: 1 in, 2 out]
        n64 = control-ref of="1"() -> (w138:refnum<vi>)
        n65 = control-ref of="2"() -> (w137:refnum<vi>)
        n66 = control-ref of="3"() -> (w136:refnum<vi>)
        n67 = control-ref of="4"() -> (w135:refnum<vi>)
        n68 = control-ref of="5"() -> (w134:refnum<vi>)
        n69 = control-ref of="6"() -> (w133:refnum<vi>)
        n70 = control-ref of="7"() -> (w132:refnum<vi>)
        n71 = control-ref of="8"() -> (w131:refnum<vi>)
        n72 = control-ref of="9"() -> (w130:refnum<vi>)
        n73 = control-ref of="10"() -> (w129:refnum<vi>)
        n74 = Build Array(w138, w137, w136, w135, w134, w133, w132, w131, w130, w129) -> (w125:refnum<vi>[])
        n75 = call "Station_Wise_Enable_Disable_Para_Indi.vi"("Communication Status Array"=w123, "error in (no error)"=w127, 10:w128, "Parameter array"=w125) -> ("error out"=w126:errorcluster, "Communication Status Array Out"=w122:string[], "Parameter array out"=w124:refnum<vi>[])  [unwired: 5 in]
        n76 = control-ref of="MACHINE 1"() -> (w157:refnum<vi>)
        n77 = control-ref of="MACHINE 2"() -> (w156:refnum<vi>)
        n78 = control-ref of="MACHINE 3"() -> (w155:refnum<vi>)
        n79 = control-ref of="MACHINE 4"() -> (w154:refnum<vi>)
        n80 = control-ref of="MACHINE 5"() -> (w153:refnum<vi>)
        n81 = control-ref of="MACHINE 6"() -> (w152:refnum<vi>)
        n82 = control-ref of="MACHINE 7"() -> (w149:refnum<vi>)
        n83 = control-ref of="MACHINE 8"() -> (w148:refnum<vi>)
        n84 = control-ref of="MACHINE 9"() -> (w147:refnum<vi>)
        n85 = control-ref of="MACHINE 10"() -> (w146:refnum<vi>)
        n86 = control-ref of="Autonomous Check Points Press"() -> (w144:refnum<vi>)
        n87 = Build Array(w157, w156, w155, w154, w153, w152, w149, w148, w147, w146) -> (w145:refnum<vi>[])
        n88 = call "Station_Wise_Enable_Disable_Alalrm_Indi.vi"("Autonomous Check Points Press"=w144, "error in (no error)"=w126, 10:w128, "Alarm array"=w145) -> ("error out"=w143:errorcluster, "Valid Indicators"=w142:refnum<vi>[])  [unwired: 6 in]
        n89 = Bundle By Name(cluster=w128, "Reading"=w124, "Shift Time stamp"=w141, "Com Status Station"=w122, "ALARAM INDICATOR REF"=w142) -> (w151:T13)
      }
      frame "Int_3" {
        w174 = string[] ["MACHINE_NAME", "RECIPE_NAME", "RECIPE_NUMBER", "Top_zone_1_Max", "Top_zone_1_Min", "Top_zone_2_Max", "Top_zone_2_Min", "Top_zone_3_Max", "Top_zone_3_Min", "Top_zone_4_Max", "Top_zone_4_Min", "Top_zone_5_Max", "Top_zone_5_Min", "Top_zone_6_Max", "Top_zone_6_Min", "Top_zone_7_Max", "Top_zone_7_Min", "Top_zone_8_Max", "Top_zone_8_Min", "Bottom_zone_1_Max", "Bottom_zone_1_Min", "Bottom_zone_2_Max", "Bottom_zone_2_Min", "Bottom_zone_3_Max", "Bottom_zone_3_Min", "Bottom_zone_4_Max", "Bottom_zone_4_Min", "Bottom_zone_5_Max", "Bottom_zone_5_Min", "Bottom_zone_6_Max", "Bottom_zone_6_Min", "Bottom_zone_7_Max", "Bottom_zone_7_Min", "Bottom_zone_8_Max", "Bottom_zone_8_Min", "Heating_time_Max", "Heating_time_Min"]  # columns
        # "read parameteres at first"
        n90 = Unbundle By Name(w189) -> ("SQL reference"=w191:T14)
        n91 = call <vilib>:"DB Tools Select Data.vi"("condition"="", "error in (no error)"=w187, "columns"=string[] ["MR_RETURN_TIMERS_MAX", "MR_RETURN_TIMERS_MIN", "HOLDING_TIMERS_MAX", "HOLDING_TIMERS_MIN", "PRESSURE_1ST_MAX", "PRESSURE_1ST_MIN", "PRESSURE_2ND_MAX", "PRESSURE_2ND_MIN", "MACHINE_NAME", "RECIPE_NAME", "RECIPE_NUMBER"] ("String"), "table"="dbo.PARAMETERS", "connection reference"=w191) -> ("error out"=w197:errorcluster, "data"=w196:variant[][], "connection reference out"=w177:T14)  [unwired: 1 in]
        n92 = Variant To Data(error in=w197, type=string[][] [[""]], Variant=w196) -> (data=w188:string[][], error out=w194:errorcluster)
        n93 = call <vilib>:"Clear Errors.vi"("error in (no error)"=w194) -> ("error out"=w179:errorcluster)  [unwired: 5 in, 1 out]
        n94 = Bundle By Name(cluster=w189, "Read Parameteres"=w188) -> (w186:T13)
        n95 = call <vilib>:"DB Tools Select Data.vi"("condition"="", "error in (no error)"=w179, "columns"=w174, "table"="dbo.OVEN_PARAMETERS", "connection reference"=w177) -> ("error out"=w180:errorcluster, "data"=w181:variant[][], "connection reference out"=w176:T14)  [unwired: 1 in]
        n96 = Variant To Data(error in=w180, type=string[][] [[""]], Variant=w181) -> (data=w175:string[][], error out=w183:errorcluster)
        n97 = call <vilib>:"Clear Errors.vi"("error in (no error)"=w183) -> ("error out"=w178:errorcluster)  [unwired: 5 in, 1 out]
        n98 = Bundle By Name(cluster=w186, "SQL reference"=w176, "Oven Read Parameteres"=w175) -> (w185:T13)
      }
      frame "BUTTON_SWITCH" {
        # "Logic to shuful Screen tab 20 Sec"
        n99 = call "Elapsed Time"() -> ("Time has Elapsed"=w203:bool)  [unwired: 12 in, 7 out]
        n100 = case shown="True" w203 {
          frame False {
          }
          frame True {
            w212 = T17 [enum."T.F. GROUP 1", enum."T.F. GROUP 2", enum."AUTO CHECK", enum."T.F. PARA", enum."OVEN PARA 1", enum."OVEN PARA 2"] items=["T.F. GROUP 1", "T.F. GROUP 2", "AUTO CHECK", "T.F. PARA", "OVEN PARA 1", "OVEN PARA 2"] ("Tab Control")
            n101 = feedback #1(0) -> (w213:i32)
            n102 = Increment(x=w213) -> (x+1=w208:i32)
            n103 = Array Size(array=w212) -> (size(s)=w211:i32)
            n104 = Greater Or Equal?(x=w208, y=w211) -> (x >= y?=w210:bool)
            n105 = Index Array(array=w212, index=w213) -> (element=w206:T2)
            n106 = Select(t=0, s=w210, f=w208) -> (s? t:f=w207:i32)
            n107 = feedback-in #1(w207) -> ()
            n108 = property on="Tab Control" class="TabCtl (strict)"("Value"=w206) -> ()  [unwired: 2 in, 2 out]
          }
        }
        n109 = case shown="False" "Close" {
          tunnel: [Station_wise_live_breakdown_loop."PLC_com" Station_wise_live_breakdown_loop."STOP"] -> w204
          tunnel: [FALSE TRUE] -> w202
          tunnel: w201 -> [w215 w218]
          tunnel: [w215 w218] -> w200
          frame False {
          }
          frame True {
          }
        }
      }
      frame "PLC_com", Default {
        (unwired) "SELECT %s from CON_STATUS WHERE Sr_No = 1 " ("SQL query")
        # "PLC Communication Indicator Update and  and timer/pressure values"
        n110 = Unbundle By Name(w222) -> ("Indicator refrence"=w230:refnum<vi>[], "SQL reference"=w232:T14, "Station Number"=w231:string[], "Reading"=w223:refnum<vi>[])
        n111 = for {
          tunnel: w231 -> [w245] mode=indexing
          tunnel: w232 -> [w266]
          tunnel: w230 -> [w264] mode=indexing
          tunnel: w229 -> [w249]
          tunnel: [w258] -> w227
          tunnel: [w253] -> _ mode=indexing
          tunnel: [w260] -> _ mode=indexing
          tunnel: w223 -> [w247] mode=indexing
          shift-right: [w246] -> w221
          shift-left: w222 -> [w246]
          w255 = 5  # dimension size
          w275 = 0 ("index (row)")
          # "Communication Indicator"
          # "Timer/pressure values"
          n112 = call <vilib>:"Trim Whitespace.vi"("string"=w245) -> ("trimmed string"=w244:string)  [unwired: 1 in]
          n113 = Format Into String(format string="SELECT T%s from CON_STATUS" ("SQL query"), w244) -> (resulting string=w274:string)  [unwired: 2 in, 1 out]
          n114 = call-poly <vilib>:"DB Tools Execute Query.vi"("error in (no error)"=w249, "SQL query"=w274, "connection reference"=w266) -> ("error out"=w276:errorcluster, "recordset reference"=w271:T16)  [unwired: 5 in]
          n115 = call-poly <vilib>:"DB Tools Fetch Recordset Data.vi"("error in (no error)"=w276, "recordset reference"=w271) -> ("error out"=w277:errorcluster, "recordset data"=w273:variant[][], "recordset reference out"=w272:T16)  [unwired: 3 in]
          n116 = call "VARIENT_TO_DATA.vi"("data"=w273, "error in (no error)"=w277) -> ("Table"=w253:string[][], "error out"=w263:errorcluster)  [unwired: 7 in]
          n117 = call-poly <vilib>:"DB Tools Free Object.vi"("recordset reference"=w272) -> ()  [unwired: 9 in, 2 out]
          n118 = call <vilib>:"Clear Errors.vi"("error in (no error)"=w263) -> ("error out"=w262:errorcluster)  [unwired: 5 in, 1 out]
          n119 = Index Array(array=w253, index (row)=w275, index (col)=w275) -> (element=w260:string)
          n120 = property on="Property Node" class="Clust"(reference=w264, error in=w262) -> (reference out=w257:refnum<vi>, error out=w261:errorcluster, "Controls[]"=w268:refnum<vi>[])
          n121 = Reshape Array(w253, w255) -> (w254:string[])
          n122 = Decimal String To Number(string=w260) -> (number=w242:i32)  [unwired: 2 in, 1 out]
          n123 = Fract/Exp String To Number(string=w254) -> (number=w252:dbl[])  [unwired: 3 in, 1 out]
          n124 = Not Equal To 0?(x=w242) -> ()  [unwired: 1 out]
          n125 = control-ref of="String Indicator 8"() -> (w267:refnum<vi>)
          n126 = Index Array(array=w268, index=4) -> (element=w270:refnum<vi>)
          n127 = To More Specific Class(target class=w267, reference=w270, error in=w261) -> (specific class reference=w243:refnum<vi>, error out=w241:errorcluster)
          n128 = Delete From Array(array=w252, index=0) -> (array with subset deleted=w248:dbl[])  [unwired: 1 in, 1 out]
          n129 = Array To Cluster(array=w248) -> (cluster=w250:T18)
          n130 = case shown="1" w242 {
            tunnel: w243 -> [w282 w287]
            tunnel: [w280 w285] -> w239
            tunnel: w241 -> [w279 w284]
            tunnel: [w278 w283] -> w240
            frame 0, Default {
              w281 = FALSE
              n131 = property on="Property Node" class="Bool (strict)"(reference=w282, error in=w279, "Blinking"=w281, "Value"=w281) -> (reference out=w278:refnum<vi>, error out=w280:errorcluster)
            }
            frame 1 {
              w286 = TRUE
              n132 = property on="Property Node" class="Bool (strict)"(reference=w287, error in=w284, "Blinking"=w286, "Value"=w286) -> (reference out=w283:refnum<vi>, error out=w285:errorcluster)
            }
          }
          n133 = property on="Property Node" class="Clust (strict)"(reference=w247, "Value"=w250) -> ()  [unwired: 1 in, 2 out]
          n134 = Wait (ms)(milliseconds to wait=u32 100) -> ()  [unwired: 1 out]
          n135 = Build Array(w257, w240) -> (w256:refnum<vi>[])
          n136 = for {
            tunnel: [w290] -> w258
            tunnel: w256 -> [w289] mode=indexing
            tunnel: w239 -> [w288]
            n137 = call <vilib>:"Clear Errors.vi"("error in (no error)"=w288) -> ("error out"=w292:errorcluster)  [unwired: 5 in, 1 out]
            n138 = Close Reference(reference=w289, error in (no error)=w292) -> (error out=w291:errorcluster)
            n139 = call <vilib>:"Clear Errors.vi"("error in (no error)"=w291) -> ("error out"=w290:errorcluster)  [unwired: 5 in, 1 out]
          }
        }
        n140 = local read "Close"() -> (w228:bool)
        n141 = case shown="False" w228 {
          tunnel: [Station_wise_live_breakdown_loop."Alaram_stat" Station_wise_live_breakdown_loop."STOP"] -> w225
          tunnel: [FALSE TRUE] -> w224
          tunnel: w227 -> [w233 w236]
          tunnel: [w233 w236] -> w226
          frame False {
          }
          frame True {
          }
        }
      }
      frame "Alaram_stat" {
        # "alarm"
        n142 = Unbundle By Name(w295) -> ("ALARAM INDICATOR REF"=w315:refnum<vi>[], "SQL reference"=w312:T14, "Station Number"=w304:string[])
        n143 = call-poly <vilib>:"DB Tools Execute Query.vi"("error in (no error)"=w294, "SQL query"="ALARM_STATUS", "connection reference"=w312) -> ("error out"=w307:errorcluster, "recordset reference"=w306:T16)  [unwired: 5 in]
        n144 = call-poly <vilib>:"DB Tools Fetch Recordset Data.vi"("error in (no error)"=w307, "recordset reference"=w306) -> ("error out"=w309:errorcluster, "recordset data"=w310:variant[][], "recordset reference out"=w305:T16)  [unwired: 3 in]
        n145 = call "VARIENT_TO_DATA.vi"("data"=w310, "error in (no error)"=w309) -> ("Table"=w311:string[][], "error out"=w300:errorcluster)  [unwired: 7 in]
        n146 = Decimal String To Number(string=w304) -> (number=w303:i32[])  [unwired: 2 in, 1 out]
        n147 = Index Array(array=w311, index (row)=0) -> (element=w302:string[])  [unwired: 1 in]
        n148 = call-poly <vilib>:"DB Tools Free Object.vi"("error in (no error)"=w300, "recordset reference"=w305) -> ("error out"=w293:errorcluster)  [unwired: 8 in, 1 out]
        n149 = for {
          tunnel: w302 -> [w324]
          tunnel: w303 -> [w322] mode=indexing
          tunnel: [w323] -> w301 mode=indexing
          n150 = Decrement(x=w322) -> (x-1=w321:i32)
          n151 = Index Array(array=w324, index=w321) -> (element=w323:string)
          n152 = Wait (ms)(milliseconds to wait=u32 20) -> ()  [unwired: 1 out]
        }
        "ALARM ARRAY" <- w301
        n153 = for {
          tunnel: w315 -> [w336] mode=indexing
          tunnel: [w326] -> w296
          tunnel: w293 -> [w337]
          tunnel: w301 -> [w335] mode=indexing
          n154 = Decimal String To Number(string=w335) -> (number=w338:i32)  [unwired: 2 in, 1 out]
          n155 = control-ref of="ALARAM CLST REF"() -> (w339:refnum<vi>)
          n156 = call <vilib>:"Clear Errors.vi"("error in (no error)"=w337) -> ("error out"=w341:errorcluster)  [unwired: 5 in, 1 out]
          n157 = Number To Boolean Array(number=w338) -> (Boolean array=w332:bool[])
          n158 = property on="Property Node" class="Clust"(reference=w336, error in=w341) -> (reference out=w325:refnum<vi>, error out=w340:errorcluster, "Controls[]"=w342:refnum<vi>[])
          n159 = Split 1D Array(array=w332, index=8) -> (first subarray=w330:bool[])  [unwired: 1 out]
          n160 = And Array Elements(Boolean array=w330) -> (logical AND=w329:bool)
          n161 = Build Array (concatenate)(w330, w329) -> (w331:bool[])
          n162 = for {
            N: 9 -> [_]
            tunnel: w342 -> [w353]
            tunnel: w339 -> [w349]
            tunnel: w331 -> [w348] mode=indexing
            tunnel: w340 -> [w352]
            tunnel: [w344] -> w327
            i -> [w350]
            n163 = Index Array(array=w353, index=w350) -> (element=w354:refnum<vi>)
            n164 = To More Specific Class(target class=w349, reference=w354, error in=w352) -> (specific class reference=w355:refnum<vi>, error out=w351:errorcluster)
            n165 = property on="Property Node" class="Bool"(reference=w355, error in=w351, "Value"=w348) -> (reference out=w346:refnum<vi>, error out=w347:errorcluster)
            n166 = Close Reference(reference=w346, error in (no error)=w347) -> (error out=w345:errorcluster)
            n167 = call <vilib>:"Clear Errors.vi"("error in (no error)"=w345) -> ("error out"=w344:errorcluster)  [unwired: 5 in, 1 out]
            n168 = Wait (ms)(milliseconds to wait=u32 10) -> ()  [unwired: 1 out]
          }
          n169 = Wait (ms)(milliseconds to wait=u32 100) -> ()  [unwired: 1 out]
          n170 = Close Reference(reference=w325, error in (no error)=w327) -> (error out=w326:errorcluster)
        }
        n171 = local read "Close"() -> (w299:bool)
        n172 = case shown="False" w299 {
          tunnel: [Station_wise_live_breakdown_loop."Product_count" Station_wise_live_breakdown_loop."STOP"] -> w298
          tunnel: [FALSE TRUE] -> w297
          frame False {
          }
          frame True {
          }
        }
        n173 = call <vilib>:"Clear Errors.vi"("error in (no error)"=w296) -> ("error out"=w314:errorcluster)  [unwired: 5 in, 1 out]
      }
      frame "Product_count" {
        # "PRODUCTION VALUE"
        n174 = Unbundle By Name(w358) -> ("Product List"=w365:string[][], "Indicator refrence"=w379:refnum<vi>[], "SQL reference"=w378:T14, "Station Number"=w377:string[], "Shift Time stamp"=w375:timestamp[])
        n175 = Get Date/Time In Seconds() -> (seconds since 1Jan1904=w367:timestamp)
        n176 = Unbundle By Name(w358) -> ("Reading"=w359:refnum<vi>[])
        n177 = call "Timestamp to string.vi"("time stamp"=w367) -> ("Date"=w366:string)  [unwired: 8 in, 2 out]
        n178 = Get Date/Time String(seconds (now)=w367, want seconds? (F)=TRUE) -> (time string=w368:string)  [unwired: 1 in, 1 out]
        n179 = call "Get Shift.vi"("error in (no error)"=w374, "Time Stamp Out"=w375) -> ("error out"=w373:errorcluster, "Shift"=w372:i32)  [unwired: 8 in]
        n180 = call <vilib>:"Space Constant.vi"() -> ("String"=w369:string)
        n181 = Concatenate Strings(w366, w369, w368) -> (→"Date / Time : 3":string)
        n182 = for {
          tunnel: w379 -> [w426] mode=indexing
          tunnel: w378 -> [w436]
          tunnel: w377 -> [w400] mode=indexing
          tunnel: w373 -> [w435]
          tunnel: [w411] -> w363
          tunnel: w372 -> [w438]
          tunnel: w366 -> [w437]
          tunnel: w365 -> [w418]
          tunnel: w359 -> [w403] mode=indexing
          tunnel: w358 -> [w402]
          tunnel: [w399] -> w357 mode=indexing
          tunnel: [w387] -> w356 mode=indexing
          i -> [w401]
          # "Ned to update this"
          n183 = Format Into String(format string="SELECT \n  PRODUCTION_COUNT,PRODUCT_CODE \nFROM ST%S_PRODUCTION_COUNT\nWHERE LOG_ID = (SELECT MAX(LOG_ID) FROM ST%S_PRODUCTION_COUNT) AND SHIFT = %d AND PLAN_DATE = '%S' " ("SQL query"), w400, w400, w438, w437) -> (resulting string=w386:string)  [unwired: 2 in, 1 out]
          n184 = Decimal String To Number(string=w400) -> (number=w417:i32)  [unwired: 2 in, 1 out]
          n185 = Decrement(x=w417) -> (x-1=w416:i32)
          n186 = Index Array(array=w418, index (row)=w416) -> (element=w415:string[])  [unwired: 1 in]
          n187 = call "Execute query.vi"("error in (no error)"=w435, "String"=w386, "connection reference"=w436) -> ("error out"=w425:errorcluster, "Table"=→"Table":string[][], "ACTUAL  PLC PRODUCT CODE"=w392:i32, "ACTUAL  PLC COUNT"=w398:i32)  [unwired: 3 in, 2 out]
          "ACTUAL  PLC COUNT" <- w398
          n188 = call "Parameter_check.vi"("Machine_Number"=w400, "reference"=w403, "index"=w401, "ACTUAL  PLC PRODUCT CODE"=w392, "Cluster"=w402) -> ("out of range ?"=w387:bool)  [unwired: 5 in, 1 out]
          n189 = Decrement(x=w392) -> (x-1=w413:i32)
          n190 = property on="Property Node" class="Clust"(reference=w426, error in=w425) -> (reference out=w410:refnum<vi>, error out=w420:errorcluster, "Controls[]"=w433:refnum<vi>[])
          n191 = Index Array(array=w415, index=w413) -> (element=w414:string)
          n192 = Index Array(array=w433, index #1=2 ("index"), index #2=5 ("index"), index #3=6 ("index")) -> (element #1=w431:refnum<vi>, element #2=w429:refnum<vi>, element #3=w395:refnum<vi>)
          n193 = control-ref of="Production Count 7"() -> (w422:refnum<vi>)
          n194 = To More Specific Class(target class=w422, reference=w431, error in=w420) -> (specific class reference=w430:refnum<vi>, error out=w419:errorcluster)
          n195 = Bundle(w400, "ACTUAL  PLC PRODUCT CODE"=w392) -> (w399:cluster{string, "ACTUAL  PLC PRODUCT CODE":i32})  [unwired: 1 in]
          n196 = property on="Property Node" class="DigNum (strict)"(reference=w430, error in=w419, "Value"=w398) -> (reference out=w405:refnum<vi>, error out=w424:errorcluster)
          n197 = control-ref of="Product code"() -> (w421:refnum<vi>)
          n198 = To More Specific Class(target class=w421, reference=w429, error in=w424) -> (specific class reference=w427:refnum<vi>, error out=w423:errorcluster)
          n199 = property on="Property Node" class="Str"(reference=w427, error in=w423, "Value"=w414) -> (reference out=w408:refnum<vi>, error out=w404:errorcluster)
          n200 = control-ref of="Recipe Number"() -> (w397:refnum<vi>)
          n201 = call <vilib>:"Clear Errors.vi"("error in (no error)"=w404) -> ("error out"=w409:errorcluster)  [unwired: 5 in, 1 out]
          n202 = Close Reference(reference=w408, error in (no error)=w409) -> (error out=w406:errorcluster)
          n203 = call <vilib>:"Clear Errors.vi"("error in (no error)"=w406) -> ("error out"=w407:errorcluster)  [unwired: 5 in, 1 out]
          n204 = Close Reference(reference=w405, error in (no error)=w407) -> (error out=w389:errorcluster)
          n205 = call <vilib>:"Clear Errors.vi"("error in (no error)"=w389) -> ("error out"=w388:errorcluster)  [unwired: 5 in, 1 out]
          n206 = To More Specific Class(target class=w397, reference=w395, error in=w388) -> (specific class reference=w394:refnum<vi>, error out=w393:errorcluster)
          n207 = property on="Property Node" class="DigNum (strict)"(reference=w394, error in=w393, "Value"=w392) -> (error out=w391:errorcluster)  [unwired: 1 out]
          n208 = call <vilib>:"Clear Errors.vi"("error in (no error)"=w391) -> ("error out"=w390:errorcluster)  [unwired: 5 in, 1 out]
          n209 = Close Reference(reference=w410, error in (no error)=w390) -> (error out=w411:errorcluster)
          n210 = Wait (ms)(milliseconds to wait=u32 250) -> ()  [unwired: 1 out]
          "String" <- w400
          "Product List 2" <- w418
        }
        "Product Code/" <- w357
        n211 = local read "Close"() -> (w364:bool)
        n212 = case shown="False" w364 {
          tunnel: [Station_wise_live_breakdown_loop."Rejection_count" Station_wise_live_breakdown_loop."STOP"] -> w361
          tunnel: [FALSE TRUE] -> w360
          tunnel: w363 -> [w380 w383]
          tunnel: [w380 w383] -> w362
          frame False {
          }
          frame True {
          }
        }
        n213 = call "Email_Sender_for_Out_off_range.vi"("Out of range ?"=w356, "Product Code/"=w357) -> ()  [unwired: 9 in, 1 out]
        n214 = call <vilib>:"Clear Errors.vi"("error in (no error)"=w362) -> ("error out"=w376:errorcluster)  [unwired: 5 in, 1 out]
      }
      frame "Rejection_count" {
        # "REJECTION VALUE"
        n215 = Unbundle By Name(w455) -> ("Indicator refrence"=w459:refnum<vi>[], "SQL reference"=w458:T14, "Station Number"=w457:string[], "Shift Time stamp"=w454:timestamp[])
        n216 = Get Date/Time In Seconds() -> (seconds since 1Jan1904=w446:timestamp)
        n217 = call "Timestamp to string.vi"("time stamp"=w446) -> ("Date"=w445:string)  [unwired: 8 in, 2 out]
        n218 = Get Date/Time String(seconds (now)=w446, want seconds? (F)=TRUE) -> (time string=w447:string)  [unwired: 1 in, 1 out]
        n219 = call "Get Shift.vi"("error in (no error)"=w453, "Time Stamp Out"=w454) -> ("error out"=w452:errorcluster, "Shift"=w451:i32)  [unwired: 8 in]
        n220 = call <vilib>:"Space Constant.vi"() -> ("String"=w448:string)
        n221 = Concatenate Strings(w445, w448, w447) -> (→"Date / Time : 4":string)
        n222 = for {
          tunnel: w459 -> [w481] mode=indexing
          tunnel: w458 -> [w488]
          tunnel: w457 -> [w476] mode=indexing
          tunnel: w452 -> [w487]
          tunnel: [w466] -> w443
          tunnel: w451 -> [w491]
          tunnel: w445 -> [w490]
          n223 = Format Into String(format string="SELECT \n  REJECTION_COUNT \nFROM STATION_%S_REJECTION_DATA\nWHERE LOG_ID = (SELECT MAX(LOG_ID) FROM STATION_%S_REJECTION_DATA) AND SHIFT = %d AND PLAN_DATE = '%S' " ("SQL query"), w476, w476, w491, w490) -> (resulting string=w489:string)  [unwired: 2 in, 1 out]
          n224 = call "Execute query.vi"("error in (no error)"=w487, "String"=w489, "connection reference"=w488) -> ("error out"=w480:errorcluster, "Table"=→"Table 2":string[][], "ACTUAL  PLC PRODUCT CODE"=→"ACTUAL  PLC PRODUCT CODE 2":i32, "ACTUAL  PLC COUNT"=w477:i32)  [unwired: 3 in, 2 out]
          "ACTUAL  PLC COUNT 2" <- w477
          n225 = property on="Property Node" class="Clust"(reference=w481, error in=w480) -> (reference out=w468:refnum<vi>, error out=w479:errorcluster, "Controls[]"=w485:refnum<vi>[])
          n226 = control-ref of="Rejection count 7"() -> (w474:refnum<vi>)
          n227 = Index Array(array=w485, index=3) -> (element=w483:refnum<vi>)
          n228 = To More Specific Class(target class=w474, reference=w483, error in=w479) -> (specific class reference=w482:refnum<vi>, error out=w478:errorcluster)
          n229 = property on="Property Node" class="DigNum (strict)"(reference=w482, error in=w478, "Value"=w477) -> (reference out=w469:refnum<vi>, error out=w467:errorcluster)
          n230 = Close Reference(reference=w469, error in (no error)=w467) -> (error out=w471:errorcluster)
          n231 = call <vilib>:"Clear Errors.vi"("error in (no error)"=w471) -> ("error out"=w470:errorcluster)  [unwired: 5 in, 1 out]
          n232 = Wait (ms)(milliseconds to wait=u32 500) -> ()  [unwired: 1 out]
          n233 = Close Reference(reference=w468, error in (no error)=w470) -> (error out=w466:errorcluster)
          "String 2" <- w476
        }
        n234 = local read "Close"() -> (w444:bool)
        n235 = case shown="False" w444 {
          tunnel: [Station_wise_live_breakdown_loop."Break_down" Station_wise_live_breakdown_loop."STOP"] -> w441
          tunnel: [FALSE TRUE] -> w440
          tunnel: w443 -> [w460 w463]
          tunnel: [w460 w463] -> w442
          frame False {
          }
          frame True {
          }
        }
        n236 = call <vilib>:"Clear Errors.vi"("error in (no error)"=w442) -> ("error out"=w456:errorcluster)  [unwired: 5 in, 1 out]
      }
      frame "Break_down" {
        n237 = Unbundle By Name(w500) -> ("Indicator refrence"=w496:refnum<vi>[], "SQL reference"=w499:T14, "Station Number"=w497:string[])
        n238 = for {
          tunnel: w499 -> [w530]
          tunnel: w501 -> [w515]
          tunnel: [w508] -> w495
          tunnel: "SELECT * FROM STATION_%S_LOG_HISTORY\nWHERE LOG_ID = (SELECT max(LOG_ID) FROM STATION_%S_LOG_HISTORY);\n\n\nSELECT TOP 1 * FROM STATION_%S_LOG_HISTORY ORDER BY LOG_ID DESC;" -> [w536]
          tunnel: w497 -> [w535] mode=indexing
          tunnel: w496 -> [w514] mode=indexing
          n239 = Format Into String(format string=w536, w535, w535, w535) -> (resulting string=w529:string)  [unwired: 2 in, 1 out]
          n240 = call-poly <vilib>:"DB Tools Execute Query.vi"("error in (no error)"=w515, "SQL query"=w529, "connection reference"=w530) -> ("error out"=w531:errorcluster, "recordset reference"=w533:T16)  [unwired: 5 in]
          n241 = call-poly <vilib>:"DB Tools Fetch Recordset Data.vi"("error in (no error)"=w531, "recordset reference"=w533) -> ("error out"=w532:errorcluster, "recordset data"=w534:variant[][], "recordset reference out"=w511:T16)  [unwired: 3 in]
          n242 = call "VARIENT_TO_DATA.vi"("data"=w534, "error in (no error)"=w532) -> ("Table"=w528:string[][], "error out"=w510:errorcluster)  [unwired: 7 in]
          n243 = call-poly <vilib>:"DB Tools Free Object.vi"("error in (no error)"=w510, "recordset reference"=w511) -> ("error out"=w509:errorcluster)  [unwired: 8 in, 1 out]
          n244 = Index Array(array=w528, index (row)=0) -> (element=w526:string[])  [unwired: 1 in]
          n245 = Index Array(array=w526, index #1=1 ("index (row)"), index #2=9 ("index (row)")) -> (element #1=w513:string, element #2=w517:string)
          n246 = Equal?(x=w517, y="0") -> (x = y?=w521:bool)
          n247 = Empty String/Path?(string/path=w517) -> (empty?=w522:bool)
          n248 = Or(x=w522, y=w521) -> (x .or. y?=w523:bool)
          n249 = Select(t=FALSE ("S"), s=w523, f=TRUE ("S")) -> (s? t:f=w516:bool)
          n250 = case shown="True" w516 {
            tunnel: w509 -> [w544 w568]
            tunnel: [w543 w559] -> w508
            tunnel: w515 -> [w553 w573]
            tunnel: w514 -> [w552 w572]
            tunnel: w513 -> [w549 _]
            frame True {
              (unwired) 0 ("index")
              # "BREAKDOWN OCCURE"
              n251 = Decimal String To Number(string=w549) -> (number=w551:i32)  [unwired: 2 in, 1 out]
              n252 = for {
                N: 5 -> [_]
                tunnel: w551 -> [w558]
                tunnel: [w555] -> w546 mode=indexing
                i -> [w556]
                n253 = Decrement(x=w558) -> (x-1=w557:i32)
                n254 = Equal?(x=w556, y=w557) -> (x = y?=w555:bool)
              }
              n255 = property on="Property Node" class="Clust"(reference=w552, error in=w553) -> (reference out=w539:refnum<vi>, error out=w545:errorcluster, "Controls[]"=w554:refnum<vi>[])
              n256 = Array To Cluster(array=w546) -> (cluster=w547:T19)
              n257 = Index Array(array=w554) -> (element=w548:refnum<vi>)  [unwired: 1 in]
              n258 = property class="Ctl"(reference=w548, error in=w545, "Value"=w547) -> (reference out=w540:refnum<vi>, error out=w538:errorcluster)
              n259 = Close Reference(reference=w540, error in (no error)=w538) -> (error out=w542:errorcluster)
              n260 = call <vilib>:"Clear Errors.vi"("error in (no error)"=w542) -> ("error out"=w541:errorcluster)  [unwired: 5 in, 1 out]
              n261 = Close Reference(reference=w539, error in (no error)=w541) -> (error out=w537:errorcluster)
              n262 = Merge Errors(w537, w544) -> (w543:errorcluster)
            }
            frame False {
              (unwired) 0 ("index")
              # "NO BREAKDOWN OCCURE"
              n263 = property on="Property Node" class="Clust"(reference=w572, error in=w573) -> (reference out=w563:refnum<vi>, error out=w569:errorcluster, "Controls[]"=w574:refnum<vi>[])
              n264 = Index Array(array=w574) -> (element=w571:refnum<vi>)  [unwired: 1 in]
              n265 = Array To Cluster(array=bool[] [FALSE, FALSE, FALSE, FALSE, FALSE]) -> (cluster=w570:T20)
              n266 = property class="Ctl"(reference=w571, error in=w569, "Value"=w570) -> (reference out=w564:refnum<vi>, error out=w562:errorcluster)
              n267 = Close Reference(reference=w564, error in (no error)=w562) -> (error out=w566:errorcluster)
              n268 = call <vilib>:"Clear Errors.vi"("error in (no error)"=w566) -> ("error out"=w565:errorcluster)  [unwired: 5 in, 1 out]
              n269 = Close Reference(reference=w563, error in (no error)=w565) -> (error out=w561:errorcluster)
              n270 = Merge Errors(w561, w568) -> (w560:errorcluster)
              n271 = call <vilib>:"Clear Errors.vi"("error in (no error)"=w560) -> ("error out"=w559:errorcluster)  [unwired: 5 in, 1 out]
            }
          }
          n272 = Wait (ms)(milliseconds to wait=u32 500) -> ()  [unwired: 1 out]
        }
        n273 = local read "Close"() -> (w494:bool)
        n274 = case shown="False" w494 {
          tunnel: [Station_wise_live_breakdown_loop."Oven_Reading" Station_wise_live_breakdown_loop."STOP"] -> w493
          tunnel: [FALSE TRUE] -> w492
          tunnel: w495 -> [w502 w505]
          tunnel: [w502 w505] -> _
          frame False {
          }
          frame True {
          }
        }
      }
      frame "Oven_Reading" {
        w577 = 7  # index
        w584 = TRUE
        w596 = "9"  # Machine_Number
        w597 = "1"  # Machine_Number
        w603 = 3  # index
        w605 = 5  # index
        w607 = 4  # index
        w612 = 2  # index
        # "COM Off = YEllow\nCOM on Blinking"
        # "2nd Screen\n\n8 10.0.0.63\n9 10.0.0.75\n1 10.0.0.67"
        # "1st screen\n\n5 10.0.0.73\n4 10.0.0.71\n3 10.0.0.69\n7 10.0.0.61"
        # "Read the oven Para and compare with min max values"
        n275 = Unbundle By Name(w589) -> ("SQL reference"=w640:T14)
        n276 = call <vilib>:"DB Tools Select Data.vi"("condition"="", "error in (no error)"=w642, "table"="dbo.OVEN_CON_STATUS", "connection reference"=w640) -> ("error out"=w646:errorcluster, "data"=w647:variant[][])  [unwired: 2 in, 1 out]
        n277 = local read "Product Code/"() -> (w590:cluster{string, "ACTUAL  PLC COUNT":i32}[])
        n278 = Variant To Data(error in=w646, type=string[][] [[""]], Variant=w647) -> (data=w639:string[][], error out=w641:errorcluster)
        n279 = Index Array(array=w639, index (col) #1=4 ("disabled index (col)"), index (col) #2=3 ("index (col)"), index (col) #3=2 ("index (col)"), index (col) #4=6 ("index (col)"), index (col) #5=7 ("index (col)"), index (col) #6=8 ("index (col)"), index (col) #7=0 ("index (col)")) -> (element #1=w633:string[], element #2=w635:string[], element #3=w630:string[], element #4=w626:string[], element #5=w622:string[], element #6=w599:string[], element #7=w610:string[])  [unwired: 7 in]
        n280 = control-ref of="1 2"() -> (w632:refnum<vi>)
        n281 = control-ref of="1 3"() -> (w634:refnum<vi>)
        n282 = call "OVEN_Value_Indicator_Update.vi"("Product Code"=w590, "Cluster"=w589, "Machine_Number"="5", "Numeric"=17, "Array"=w633, "Cluster in"=w632) -> ("Boolen value of oven"=w585:bool)  [unwired: 5 in]
        n283 = control-ref of="1 4"() -> (w628:refnum<vi>)
        n284 = Split 1D Array(array=w599, index=w607) -> (first subarray=w608:string[], second subarray=w606:string[])
        n285 = call "OVEN_Value_Indicator_Update.vi"("Product Code"=w590, "Cluster"=w589, "Machine_Number"="4", "Numeric"=17, "Array"=w635, "Cluster in"=w634) -> ("Boolen value of oven"=w586:bool)  [unwired: 5 in]
        n286 = control-ref of="1 5"() -> (w625:refnum<vi>)
        n287 = Split 1D Array(array=w606, index=w605) -> (second subarray=w604:string[])  [unwired: 1 out]
        n288 = call "OVEN_Value_Indicator_Update.vi"("Product Code"=w590, "Cluster"=w589, "Machine_Number"="3", "Numeric"=17, "Array"=w630, "Cluster in"=w628) -> ("Boolen value of oven"=w587:bool)  [unwired: 5 in]
        n289 = Split 1D Array(array=w604, index=w603) -> (first subarray=w602:string[], second subarray=w600:string[])
        n290 = control-ref of="1 6"() -> (w623:refnum<vi>)
        n291 = call "OVEN_Value_Indicator_Update.vi"("Product Code"=w590, "Cluster"=w589, "Machine_Number"="7", "Numeric"=17, "Array"=w626, "Cluster in"=w625) -> ("Boolen value of oven"=w583:bool)  [unwired: 5 in]
        n292 = call "OVEN_Value_Indicator_Update.vi"("Product Code"=w590, "Cluster"=w589, "Machine_Number"="8", "Numeric"=17, "Array"=w622, "Cluster in"=w623) -> ("Boolen value of oven"=w582:bool)  [unwired: 5 in]
        n293 = Delete From Array(array=w600) -> (deleted portion=w601:string)  [unwired: 2 in, 1 out]
        n294 = Build Array (concatenate)(w608, w602, w601) -> (w598:string[])
        n295 = control-ref of="1 7"() -> (w621:refnum<vi>)
        n296 = call "OVEN_Value_Indicator_Update.vi"("Product Code"=w590, "Cluster"=w589, "Machine_Number"=w596, "Numeric"=7, "Array"=w598, "Cluster in"=w621) -> ("Boolen value of oven"=w581:bool)  [unwired: 5 in]
        n297 = control-ref of="1 8"() -> (w620:refnum<vi>)
        n298 = Split 1D Array(array=w610, index=w612) -> (first subarray=w611:string[], second subarray=w578:string[])
        n299 = Delete From Array(array=w578) -> (deleted portion=w576:string)  [unwired: 2 in, 1 out]
        n300 = Delete From Array(array=w578, index=w577) -> (deleted portion=w575:string)  [unwired: 1 in, 1 out]
        n301 = Build Array (concatenate)(w611, w575, w576) -> (w609:string[])
        n302 = call "OVEN_Value_Indicator_Update.vi"("Product Code"=w590, "Cluster"=w589, "Machine_Number"=w597, "Numeric"=3, "Array"=w609, "Cluster in"=w620) -> ("Boolen value of oven"=w588:bool)  [unwired: 5 in]
        n303 = Build Array(w588, w584, w587, w586, w585, w584, w583, w582, w581) -> (w580:bool[])
        n304 = Array To Cluster(array=w580) -> (cluster=→"OVEN STATUS AUTONOMOUS":T21)
        n305 = disable-structure shown="Disabled" {
          frame Disabled {
            n306 = call "Email_Sender_for_Out_off_range.vi"() -> ()  [unwired: 11 in, 1 out]
          }
          frame Enabled {
          }
        }
      }
      frame "STOP" {
        n307 = call "Dashboard exit vi.vi"("error in (no error)"=w649, "Exit in"=TRUE, "Enum"=enum16{"Write", "Read"}."Write") -> ("error out"=w650:errorcluster)  [unwired: 7 in, 1 out]
      }
    }
    n308 = Wait (ms)(milliseconds to wait=u32 250) -> ()  [unwired: 1 out]
    n309 = call "lopp execution time check.vi"(8:w65) -> (0:→"?":T1[], "appended array"=→"appended array":u32[])  [unwired: 9 in]
  }
  n310 = property on="Tab Control" class="TabCtl (strict)"("Tabs Visible?"=TRUE) -> ()  [unwired: 2 in, 2 out]
  n311 = disable-structure shown="Disabled" {
    frame Disabled {
      w656 = FALSE
      n312 = property on="Station Name 2" class="Bool"("Blinking"=w656) -> ()  [unwired: 2 in, 2 out]
      n313 = property on="Station Name 2" class="Bool"("Blinking"=w656) -> ()  [unwired: 2 in, 2 out]
      n314 = property on="Station Name 2" class="Bool"("Blinking"=w656) -> ()  [unwired: 2 in, 2 out]
      n315 = property on="Station Name 2" class="Bool"("Blinking"=w656) -> ()  [unwired: 2 in, 2 out]
      n316 = property on="Station Name 2" class="Bool"("Blinking"=w656) -> ()  [unwired: 2 in, 2 out]
      n317 = property on="Station Name 2" class="Bool"("Blinking"=w656) -> ()  [unwired: 2 in, 2 out]
      n318 = property on="Station Name 2" class="Bool"("Blinking"=w656) -> ()  [unwired: 2 in, 2 out]
    }
    frame Enabled {
    }
  }
  n319 = flat-sequence {
    frame #0 {
    }
  }
  n320 = call <vilib>:"Clear Errors.vi"("error in (no error)"=w11) -> ("error out"=w12:errorcluster)  [unwired: 5 in, 1 out]
  n321 = Unbundle By Name(w23) -> ("Indicator refrence"=w13:refnum<vi>[], "SQL reference"=w22:T14)
  n322 = call <vilib>:"DB Tools Close Connection.vi"("error in (no error)"=w12, "connection reference"=w22) -> ("error out"=w26:errorcluster)  [unwired: 5 in]
  n323 = call <vilib>:"Clear Errors.vi"("error in (no error)"=w26) -> ("error out"=w15:errorcluster)  [unwired: 5 in, 1 out]
  n324 = Close Reference(reference=w13, error in (no error)=w15) -> (error out=w14:errorcluster)
  n325 = call <vilib>:"Clear Errors.vi"("error in (no error)"=w14) -> ("error out"=w16:errorcluster)  [unwired: 5 in, 1 out]
  n326 = property class="App"(error in=w16) -> (error out=w25:errorcluster, "App.Kind"=w24:T15)  [unwired: 1 in, 1 out]
  n327 = case shown="\"Run Time System\"" w24 {
    tunnel: w25 -> [w657 w659]
    tunnel: [w657 w658] -> w17
    frame Default {
    }
    frame "Run Time System" {
      n328 = invoke class="VI" method="FP.Close"(error in=w659) -> (error out=w658:errorcluster)  [unwired: 2 in, 2 out]
    }
  }
  n329 = flat-sequence {
    tunnel: [w660] -> w18
    tunnel: w17 -> [w660]
    frame #0 {
      n330 = global write "Global 1.vi" "REMOVE VI"(TRUE ("REMOVE VI")) -> ()
    }
  }
  "error out" <- w18
